vi "Automated JV Measurement.vi"() -> ()   [LabVIEW 2011]
uses:
  TypeDefs/Scan settings.ctl
  TypeDefs/Settings Boolean.ctl
  TypeDefs/State Enumerate Ring.ctl
  <vilib>/Utility/file.llb/Write To Spreadsheet File (string).vi
  <vilib>/Utility/file.llb/Write To Spreadsheet File (DBL).vi
  <instrlib>/keithley_24xx/Keithley 24XX/Keithley 24XX.lvlib
panel:
  in  "Intensity/EQE off":bool
  out "Scan stopped?":bool
  out "Max P cond. cont. Lab.txt array":string[](array[string])
  out "Max P cont. Lab.txt array":string[](array[string])
  out "J-t cont. Lab.txt array":string[](array[string])
  out "J-V cond. cont. Lab.txt array":string[](array[string])
  out "J-V cont. Lab.txt array":string[](array[string])
  out "Go to neg. lim. Lab.txt array":string[](array[string])
  out "Start scan Lab.txt array":string[](array[string])
  out "Init/idle Lab.txt array":string[](array[string])
  out "Measure Lab.txt array":string[](array[string])
  out "Sample set. Lab.txt array":string[](array[string])
  out "Scan set. Lab.txt array":string[](array[string])
  out "Advanced Lab.txt array":string[](array[string])
  out "Calibrate?":bool
  out "reference (out) 4":i32=4168
  out "reference (out) 3":i32=4168
  out "reference (out) 2":i32=4168
  out "reference (out)":i32=4168
  out "Abort":bool
  in  "Tab Control":T1(tab)
  in  "Manual mode":bool
  in  "Cell Settings Array 1":T2(array[cluster])=[{"Cell Position"=1, "Cell Label"="", "Pixel to measure"=0, "Area (cm^2)"=0.0935, "Variable"="", "Variable value"="", "Scan settings in queue"=0}, {"Cell Position"=2, "Cell Label"="", "Pixel to measure"=0, "Area (cm^2)"=0.0935, "Variable"="", "Variable value"="", "Scan settings in queue"=0}, {"Cell Position"=3, "Cell Label"="", "Pixel to measure"=0, "Area (cm^2)"=0.0935, "Variable"="", "Variable value"="", "Scan settings in queue"=0}, {"Cell Position"=4, "Cell Label"="", "Pixel to measure"=0, "Area (cm^2)"=0.0935, "Variable"="", "Variable value"="", "Scan settings in queue"=0}, {"Cell Position"=5, "Cell Label"="", "Pixel to measure"=0, "Area (cm^2)"=0.0935, "Variable"="", "Variable value"="", "Scan settings in queue"=0}, {"Cell Position"=6, "Cell Label"="", "Pixel to measure"=0, "Area (cm^2)"=0.0935, "Variable"="", "Variable value"="", "Scan settings in queue"=0}, {"Cell Position"=7, "Cell Label"="", "Pixel to measure"=0, "Area (cm^2)"=0.0935, "Variable"="", "Variable value"="", "Scan settings in queue"=0}, {"Cell Position"=8, "Cell Label"="", "Pixel to measure"=0, "Area (cm^2)"=0.0935, "Variable"="", "Variable value"="", "Scan settings in queue"=0}, {"Cell Position"=9, "Cell Label"="", "Pixel to measure"=0, "Area (cm^2)"=0.0935, "Variable"="", "Variable value"="", "Scan settings in queue"=0}, {"Cell Position"=10, "Cell Label"="", "Pixel to measure"=0, "Area (cm^2)"=0.0935, "Variable"="", "Variable value"="", "Scan settings in queue"=0}, {"Cell Position"=11, "Cell Label"="", "Pixel to measure"=0, "Area (cm^2)"=0.0935, "Variable"="", "Variable value"="", "Scan settings in queue"=0}, {"Cell Position"=12, "Cell Label"="", "Pixel to measure"=0, "Area (cm^2)"=0.0935, "Variable"="", "Variable value"="", "Scan settings in queue"=0}, {"Cell Position"=13, "Cell Label"="", "Pixel to measure"=0, "Area (cm^2)"=0.0935, "Variable"="", "Variable value"="", "Scan settings in queue"=0}, {"Cell Position"=14, "Cell Label"="", "Pixel to measure"=0, "Area (cm^2)"=0.0935, "Variable"="", "Variable value"="", "Scan settings in queue"=0}, {"Cell Position"=15, "Cell Label"="", "Pixel to measure"=0, "Area (cm^2)"=0.0935, "Variable"="", "Variable value"="", "Scan settings in queue"=0}, {"Cell Position"=16, "Cell Label"="", "Pixel to measure"=0, "Area (cm^2)"=0.0935, "Variable"="", "Variable value"="", "Scan settings in queue"=0}] {"Scan settings in queue" items=["Default_Inv", "Default_Std", "Solarprint", "StandardJV", "TEST_std", "Test_Manual_JV_Jt_mppt", "Test_inv", "Test_inv2", "Test_inv3", "Test_inv4", "Test_inv_mpp", "Test_inv_mppt", "Test_inv_mppt_Jt", "Test_std_2", "Test_std_3", "Test_std_4", "Test_std_5"]; "Pixel to measure" items=["All", "1", "2", "3", "4", "5", "6", "7", "8"]}
  in  "Load details from file":bool
  in  "Save details to file":bool
  out "X-Y stage controller":bool
  out "PCB controller":bool
  out "Keithley 2400":bool
  in  "User Name":string
  in  "Experiment Title":string
  out "Status:":string
  in  "Move to load pos.":bool
  in  "Exit":bool
  out "Arduino":bool
  in  "Update":bool
  in  "Scan settings":T3={"J-V scan"=TRUE, "J-t scan"=FALSE, "Min voltage (V)"=0.0, "Max voltage (V)"=1.4, "Step (V)"=0.01, "Measurement delay (ms)"=10.0, "1st scan FB-SC"=TRUE, "Inverted structure"=FALSE, "Stabilisation time (s)"=0.0, "Stabilisation mode"=0, "Stabilisation value (V or A) "=0.0, "Step time (s)"=1.0, "Integration time"=0, "Repeat light scans"=FALSE, "Stabilisation in the dark?"=FALSE, "J-t Min (V)"=0.0, "J-t Max (V)"=1.4, "J-t Step (V)"=0.01, "Max. power stabilisation"=FALSE, "J-t 1st scan FB-SC"=TRUE, "J-t Inverted structure"=FALSE, "Max power tracking"=FALSE, "Vmp (V)"=0.7, "Total stabilisation time (s)"=100.0, "J-t best pixel only"=7, "Max power best pixel only"=7, "Vmp from J-V scan"=FALSE, "Intensity dependence"=FALSE, "P dep best pixel only"=7, "External quantum efficiency"=FALSE, "EQE best pixel only"=7, "WL min (nm)"=300.0, "WL max (nm)"=900.0, "WL step (nm)"=5.0, "Wait (ms)"=100.0, "No. of repeat scans"=2.0, "Only repeat for best pixel"=7, "Chopper Freq. min (Hz)"=90.0, "Time Constant min (s)"=2.0, "Stabilisation time step (s)"=1.0, "Illumination conditions"=2, "Scan rate min (V/s)"=0.1, "Scan rate max (V/s)"=1.0, "No. of scan rate steps"=1.0, "Scan rate voltage step priority"=FALSE, "Scan rate measurement delay priority"=FALSE, "J-t Illumination conditions"=0, "Chopper Freq. max (Hz)"=200.0, "No. of freq. steps"=1.0, "Time Constant max (s)"=2.0, "No. of t const. steps"=1.0, "White bias min (no. of suns)"=0.1, "White bias max (no. of suns)"=1.0, "No. of white bias steps"=1.0, "Repeat EQE scans"=FALSE, "No. of EQE scans"=2.0, "Max P stab. Specific voltage"=FALSE} {"No. of EQE scans" min=1.0 step=1.0; "No. of white bias steps" min=1.0 step=1.0; "No. of t const. steps" min=1.0 step=1.0; "Time Constant max (s)" items=["0.01s", "0.03s", "0.1s", "0.3s", "1s", "3s"]; "No. of freq. steps" min=1.0 step=1.0; "J-t Illumination conditions" items=["Light only", "Dark only", "Light then dark", "Dark then light"]; "No. of scan rate steps" min=1.0 step=1.0; "Illumination conditions" items=["Light only", "Dark only", "Light then dark", "Dark then light", "Light then dark then light", "Dark then light then dark"]; "Time Constant min (s)" items=["0.01s", "0.03s", "0.1s", "0.3s", "1s", "3s"]; "Only repeat for best pixel" items=["only for best pixel", "for best 2 pixels", "for best 3 pixels", "for best 4 pixels", "for best 5 pixels", "for best 6 pixels", "for best 7 pixels", "for all pixels"]; "No. of repeat scans" min=1.0 step=1.0; "EQE best pixel only" items=["only the best pixel", "the best 2 pixel", "the best 3 pixel", "the best 4 pixel", "the best 5 pixel", "the best 6 pixel", "the best 7 pixel", "all pixels"]; "P dep best pixel only" items=["only the best pixel", "the best 2 pixels", "the best 3 pixels", "the best 4 pixels", "the best 5 pixels", "the best 6 pixels", "the best 7 pixels", "all pixels"]; "Max power best pixel only" items=["only the best pixel", "the best 2 pixels", "the best 3 pixels", "the best 4 pixels", "the best 5 pixels", "the best 6 pixels", "the best 7 pixels", "all pixels"]; "J-t best pixel only" items=["only the best pixel", "the best 2 pixels", "the best 3 pixels", "the best 4 pixels", "the best 5 pixels", "the best 6 pixels", "the best 7 pixels", "all pixels"]; "Integration time" items=["Fast", "Normal", "High Accuracy"]; "Stabilisation mode" items=["V", "I"]; "Measurement delay (ms)" min=10.0}
  in  "Save New Settings As...":string
  in  "Check Saved Settings":u16(ring) items=["Default_Inv", "Default_Std", "Solarprint", "StandardJV", "TEST_std", "Test_Manual_JV_Jt_mppt", "Test_inv", "Test_inv2", "Test_inv3", "Test_inv4", "Test_inv_mpp", "Test_inv_mppt", "Test_inv_mppt_Jt", "Test_std_2", "Test_std_3", "Test_std_4", "Test_std_5"]
  in  "Save new settings":bool
  in  "Delete settings":bool
  out "Measurement status:":string
  out "Log Table":string[][](table)
  out "JV Curve":cluster{"Y":dbl[], "Y":dbl[]}[](graph)
  out "Number of suns":string
  in  "Stop Scan 2":bool
  in  "Start Scan":bool
  out "Finish time":timestamp caption="This experiment will finish at approximately" format="%<%H:%M:%S   %d/%m/%y>T"
  out "Time left":dbl caption="You have" format="%<%H:%M:%S>t"
  out "Measurement queue":T5(array[cluster]) {"Pixel to measure" items=["All", "1", "2", "3", "4", "5", "6", "7", "8"]}
  out "Current Angle (degrees)":dbl
  out "Pin":dbl
  out "Current (A)":dbl
  in  "Pixel":i64
  in  "Cell":i64
  in  "Shutter closed":bool
  in  "Shutter open":bool
  in  "error in (no error) 3":errorcluster
  in  "Set diode pos":bool
  in  "Go to negative limit":bool
  out "Y position":string
  out "X position":string
  in  "X -ve":bool
  in  "X +ve":bool
  in  "Y -ve":bool
  in  "Y +ve":bool
  in  "Change pin on pcb":bool
  in  "Measure current":bool
  out "File path for master log":path
  out "Experiment type":u16(ring) items=["PCB-Keithley", "PCB-EQE", "Manual-Keithley", "Manual-EQE"]
  # "Cell #"
  # "Label"
  # "Pixel #"
  # "Area (cm^2)"
  # "Variable"
  # "Variable Value"
  # "Scan Settings"
  # "Connected instruments"
  # "Label"
  # "Pixel"
  # "Condition"
  # "Jsc"
  # "Voc"
  # "PCE"
  # "FF"
  # "Vmp"
  # "to work on something else."
  # "Position"
  # "Label"
  # "Pixel"
  # "Area"
  # "Variable"
  # "Variable Value"
  # "Scan Settings"
  # "Condition"
  # "Measurement Type"
  # "Pixel Selection"
  # "Motor Control"
  # "Filter Wheel"
  # "Shutter Control"
  # "Switch board configuration"
  # "Current Measurement"
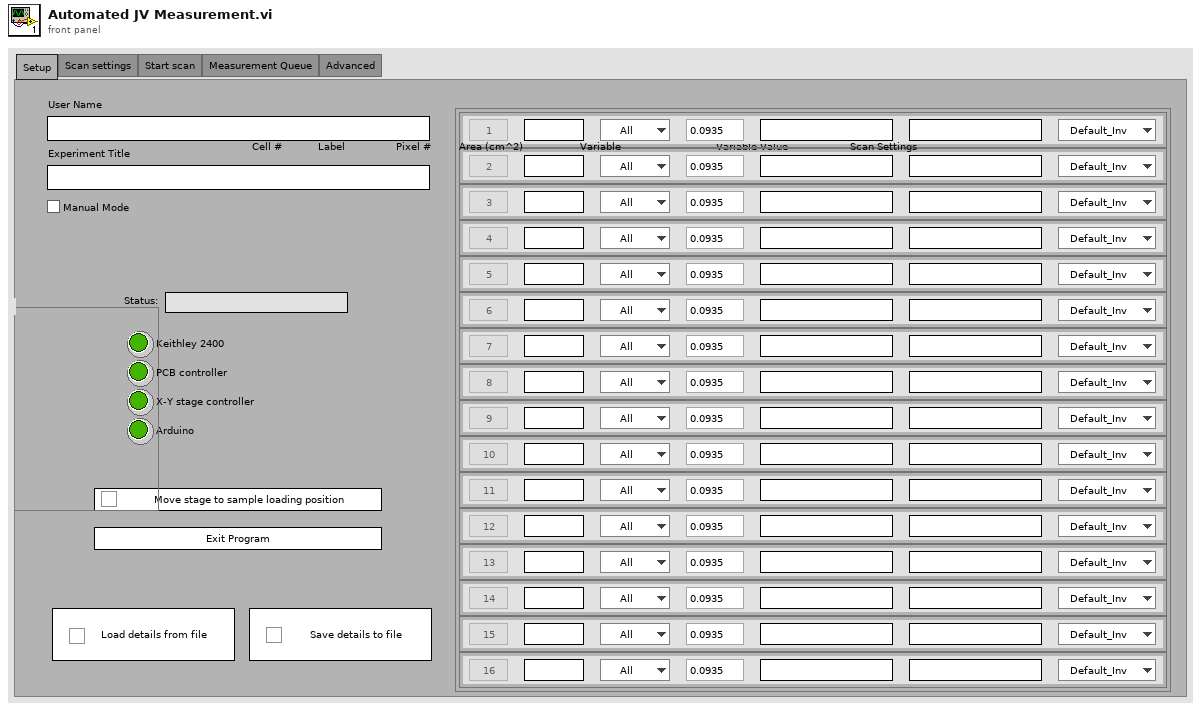
[diagram p1: front panel]
types:
  T1 = enum32{"Setup", "Scan settings", "Start scan", "Measurement Queue", "Advanced"}
  T2 = cluster{"Cell Position":i32, "Cell Label":string, "Pixel to measure":u16, "Area (cm^2)":dbl, "Variable":string, "Variable value":string, "Scan settings in queue":u16}[]
  T3 = typedef "Scan settings.ctl" = cluster{"J-V scan":T4, "J-t scan":bool, "Min voltage (V)":dbl, "Max voltage (V)":dbl, "Step (V)":dbl, "Measurement delay (ms)":dbl, "1st scan FB-SC":bool, "Inverted structure":bool, "Stabilisation time (s)":dbl, "Stabilisation mode":u16, "Stabilisation value (V or A) ":dbl, "Step time (s)":dbl, "Integration time":u16, "Repeat light scans":bool, "Stabilisation in the dark?":bool, "J-t Min (V)":dbl, "J-t Max (V)":dbl, "J-t Step (V)":dbl, "Max. power stabilisation":bool, "J-t 1st scan FB-SC":bool, "J-t Inverted structure":bool, "Max power tracking":bool, "Vmp (V)":dbl, "Total stabilisation time (s)":dbl, "J-t best pixel only":u16, "Max power best pixel only":u16, "Vmp from J-V scan":bool, "Intensity dependence":bool, "P dep best pixel only":u16, "External quantum efficiency":bool, "EQE best pixel only":u16, "WL min (nm)":dbl, "WL max (nm)":dbl, "WL step (nm)":dbl, "Wait (ms)":dbl, "No. of repeat scans":dbl, "Only repeat for best pixel":u16, "Chopper Freq. min (Hz)":dbl, "Time Constant min (s)":dbl, "Stabilisation time step (s)":dbl, "Illumination conditions":u16, "Scan rate min (V/s)":dbl, "Scan rate max (V/s)":dbl, "No. of scan rate steps":dbl, "Scan rate voltage step priority":bool, "Scan rate measurement delay priority":bool, "J-t Illumination conditions":u16, "Chopper Freq. max (Hz)":dbl, "No. of freq. steps":dbl, "Time Constant max (s)":dbl, "No. of t const. steps":dbl, "White bias min (no. of suns)":dbl, "White bias max (no. of suns)":dbl, "No. of white bias steps":dbl, "Repeat EQE scans":bool, "No. of EQE scans":dbl, "Max P stab. Specific voltage":bool}
  T4 = typedef "Settings Boolean.ctl" = bool
  T5 = cluster{"Cell Position":i32, "Cell Label":string, "Pixel to measure":u16, "Area (cm^2)":dbl, "Variable":string, "Variable value":string, "Scan settings in queue":u16, "Light or dark":string, "Measurement type":string}[]
  T6 = typedef "State Enumerate Ring.ctl" = enum16{"Initialise", "Idle", "Measure", "Notify"}
  T7 = enum8{"Enabled", "Disabled", "Disabled and Grayed Out"}
  T8 = enum16{"Left Button", "Center Button", "Right Button", "Window Close"}
  T9 = cluster{"Cell Position":i32, "Cell Label":string, "Pixel to measure":u16, "Area (cm^2)":dbl, "Variable":string, "Variable value":string, "Scan settings in queue":u16, "Light or dark":string, "Measurement type":string}
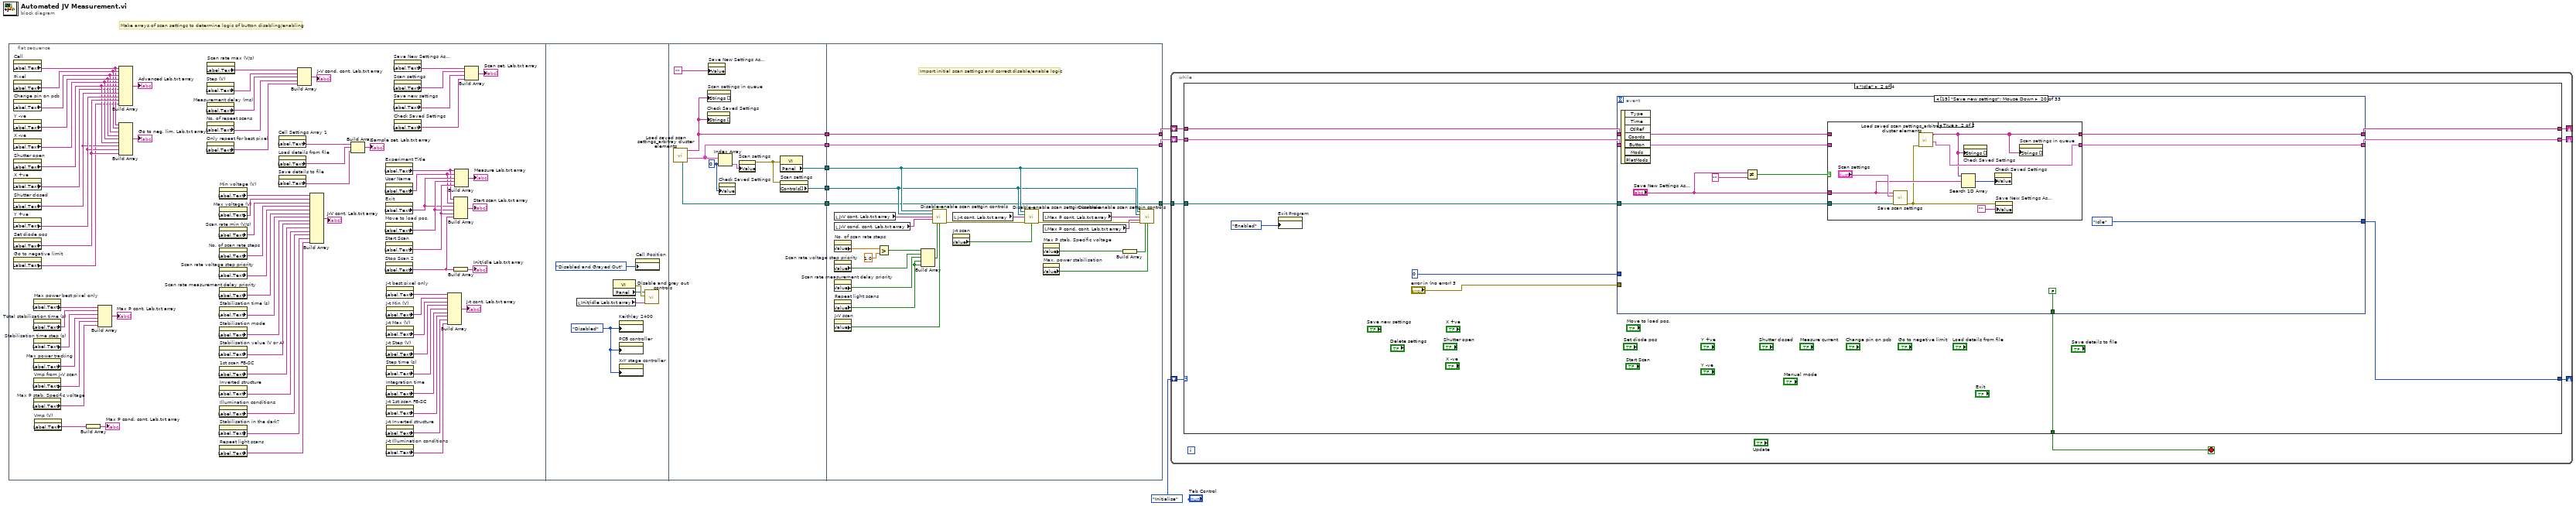
[diagram p0: block diagram]
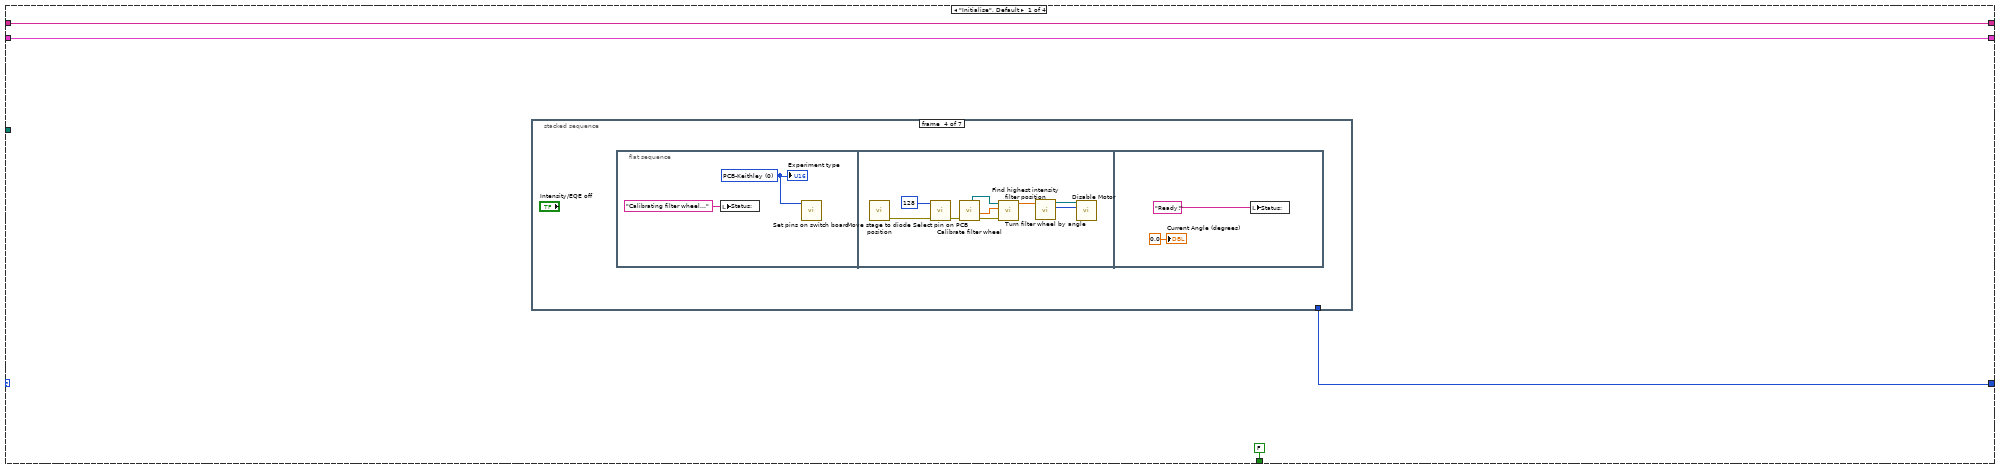
[diagram p2: hidden frame]
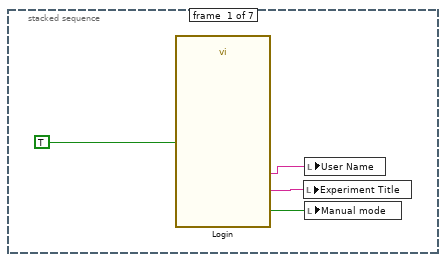
[diagram p3: hidden frame]
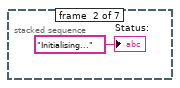
[diagram p4: hidden frame]
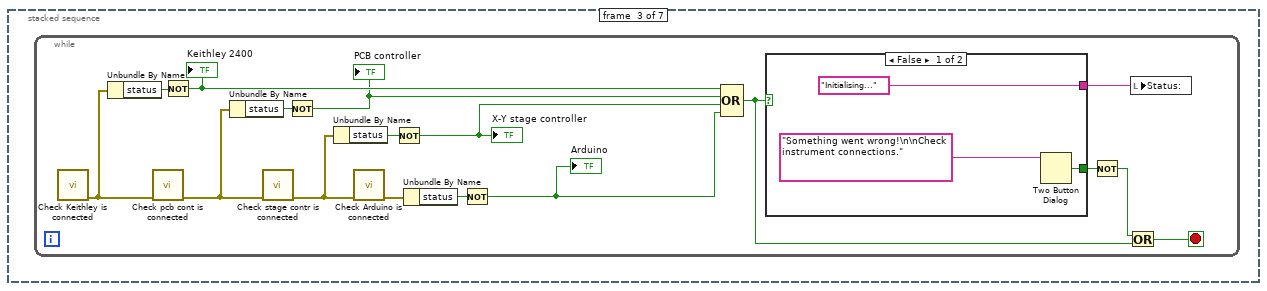
[diagram p5: hidden frame]
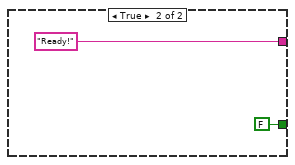
[diagram p6: hidden frame]
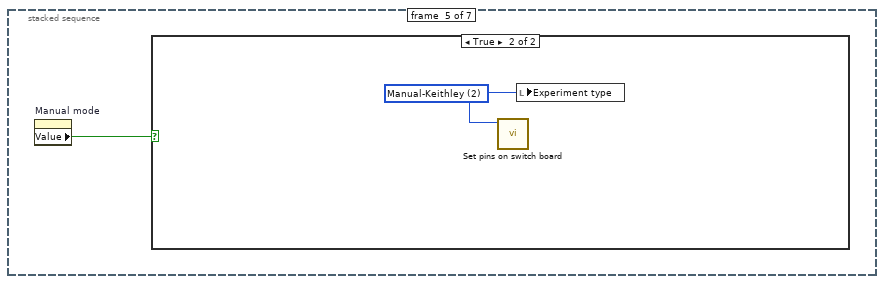
[diagram p7: hidden frame]
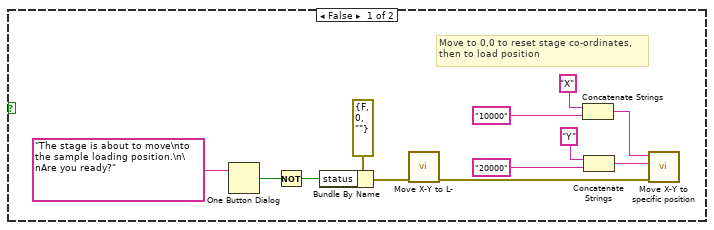
[diagram p8: hidden frame]
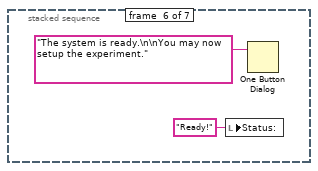
[diagram p9: hidden frame]
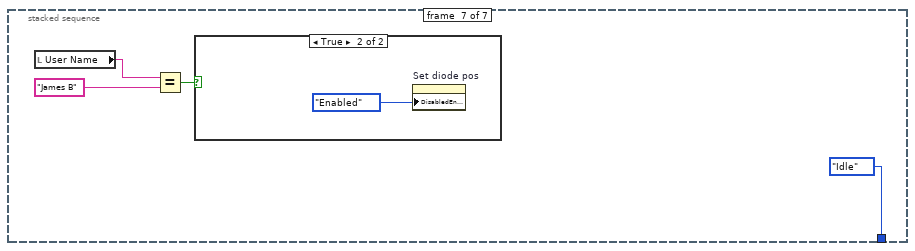
[diagram p10: hidden frame]
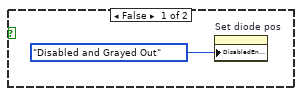
[diagram p11: hidden frame]
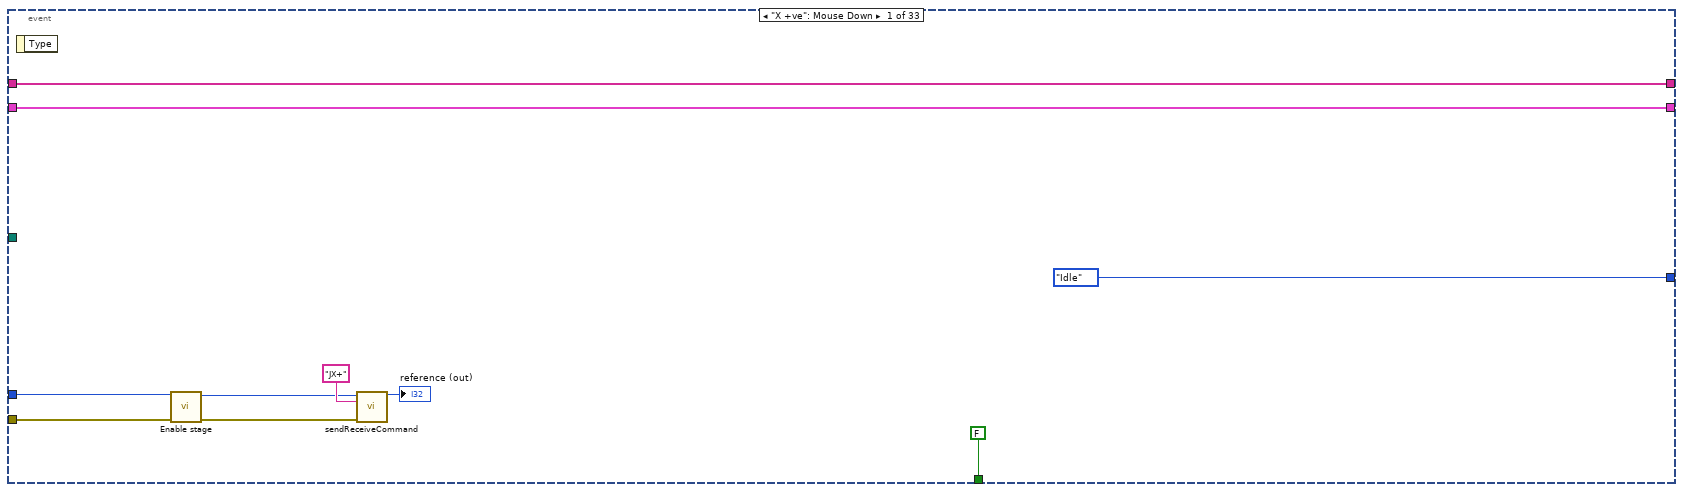
[diagram p12: hidden frame]
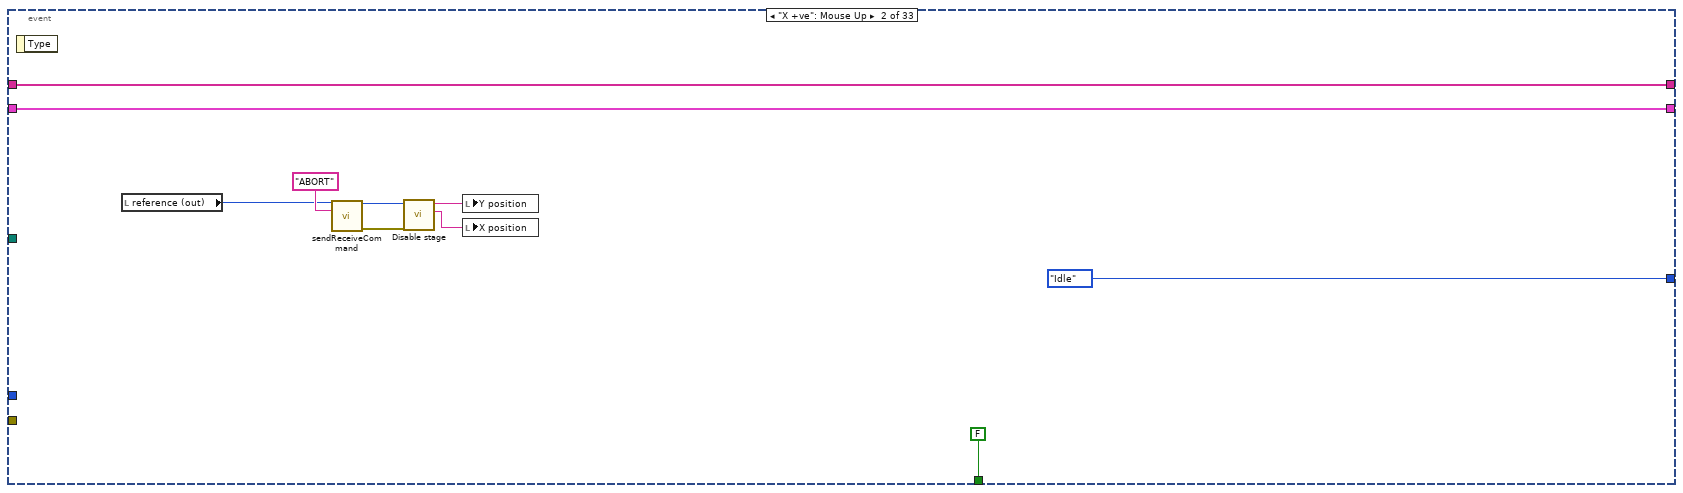
[diagram p13: hidden frame]
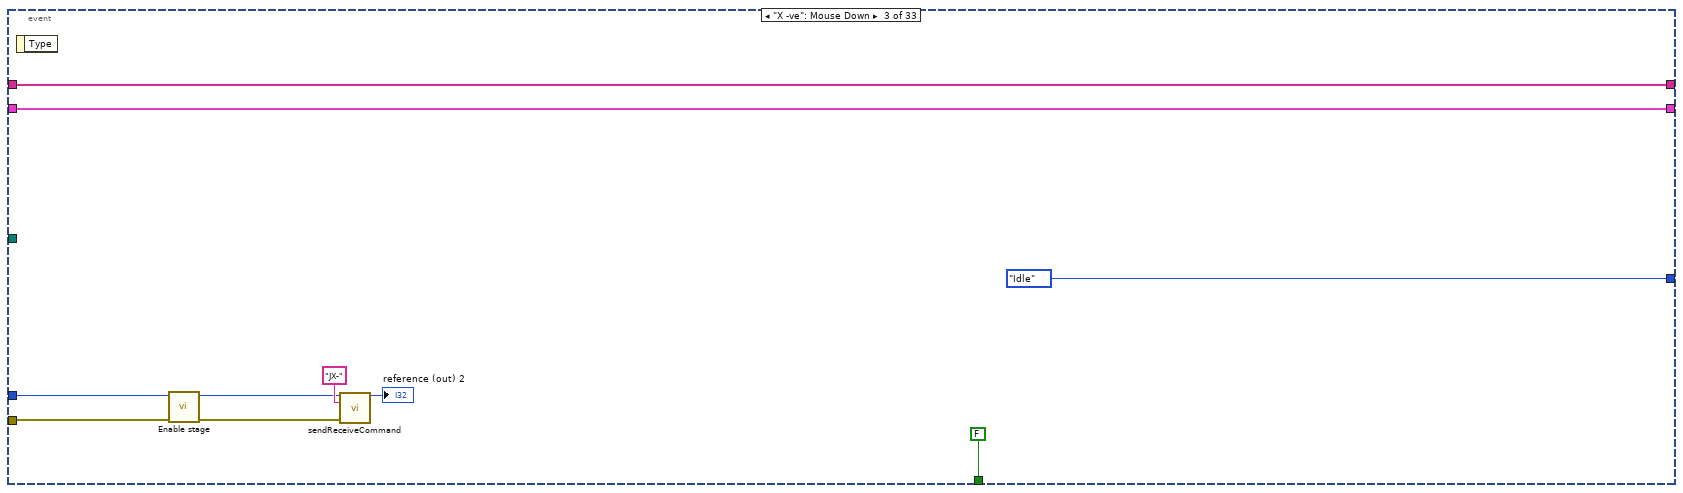
[diagram p14: hidden frame]
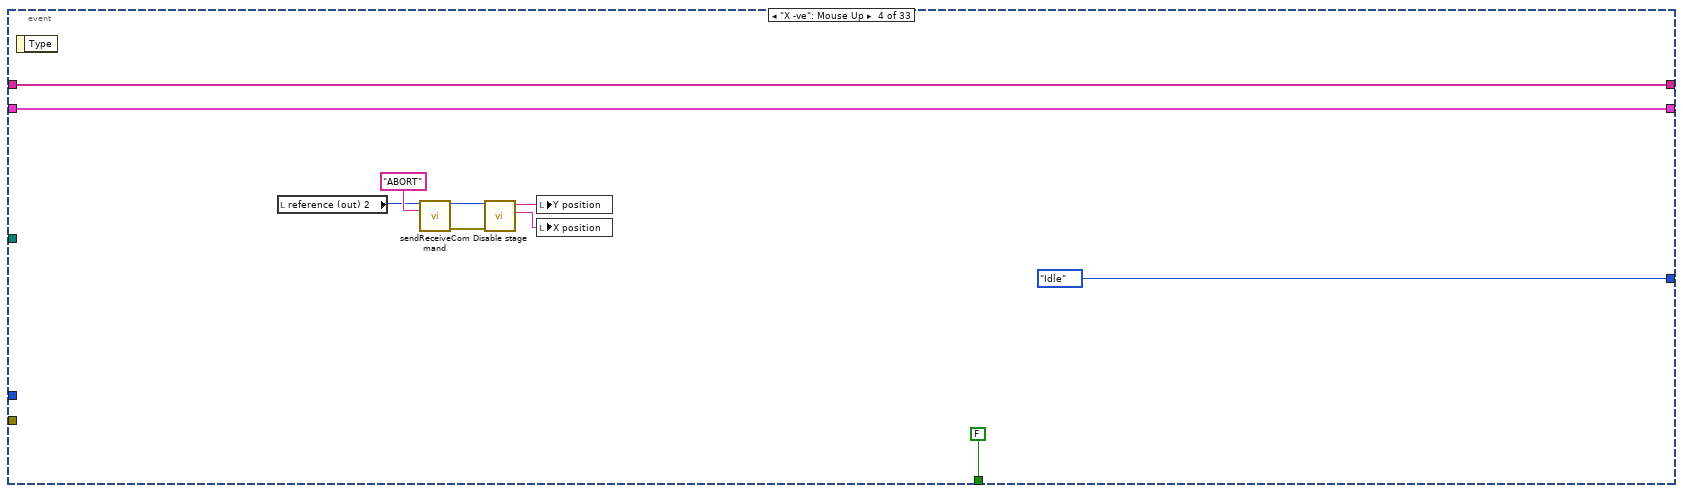
[diagram p15: hidden frame]
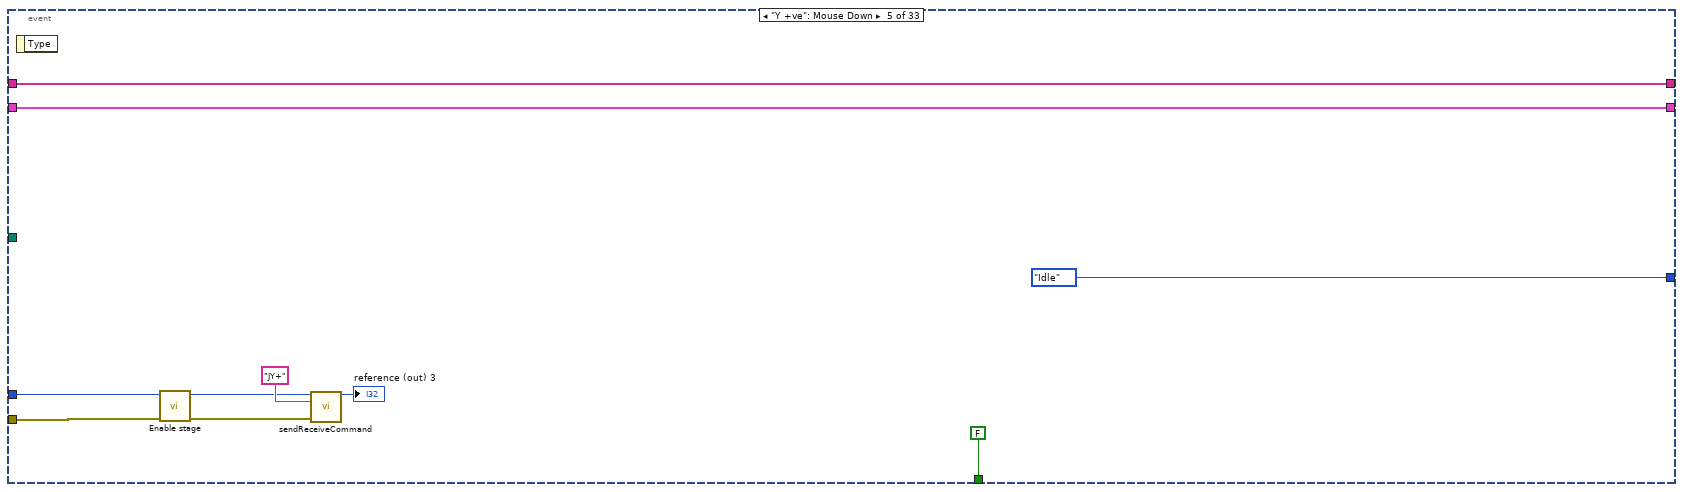
[diagram p16: hidden frame]
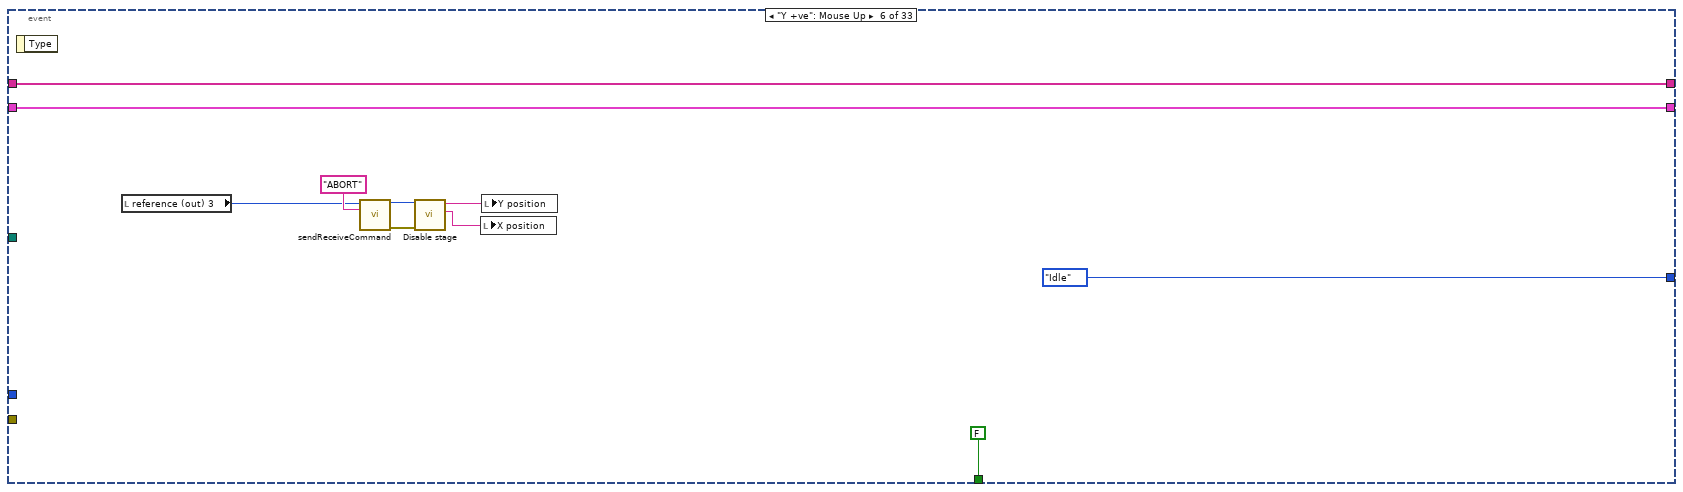
[diagram p17: hidden frame]
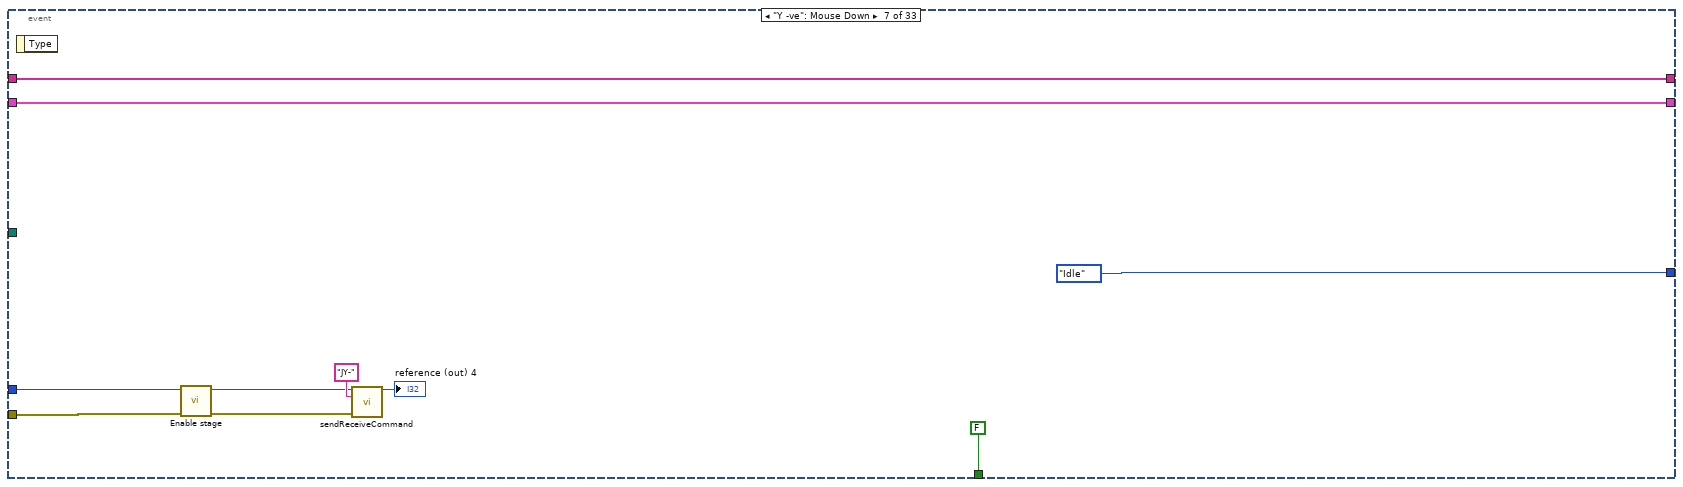
[diagram p18: hidden frame]
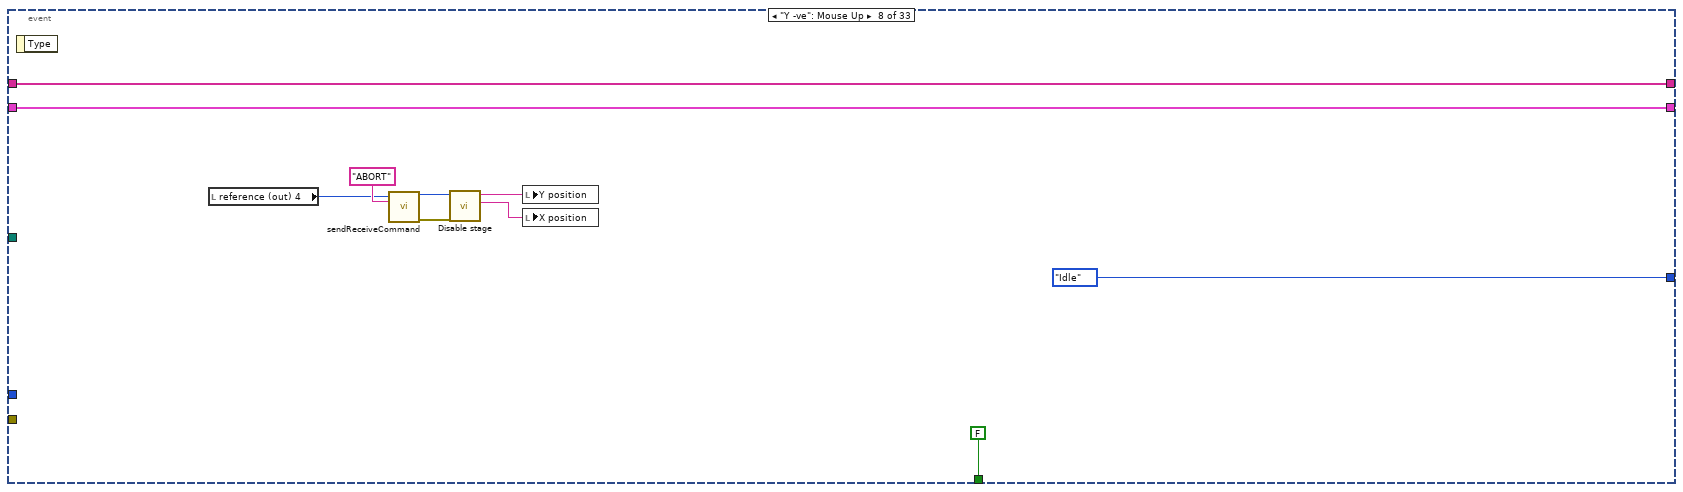
[diagram p19: hidden frame]
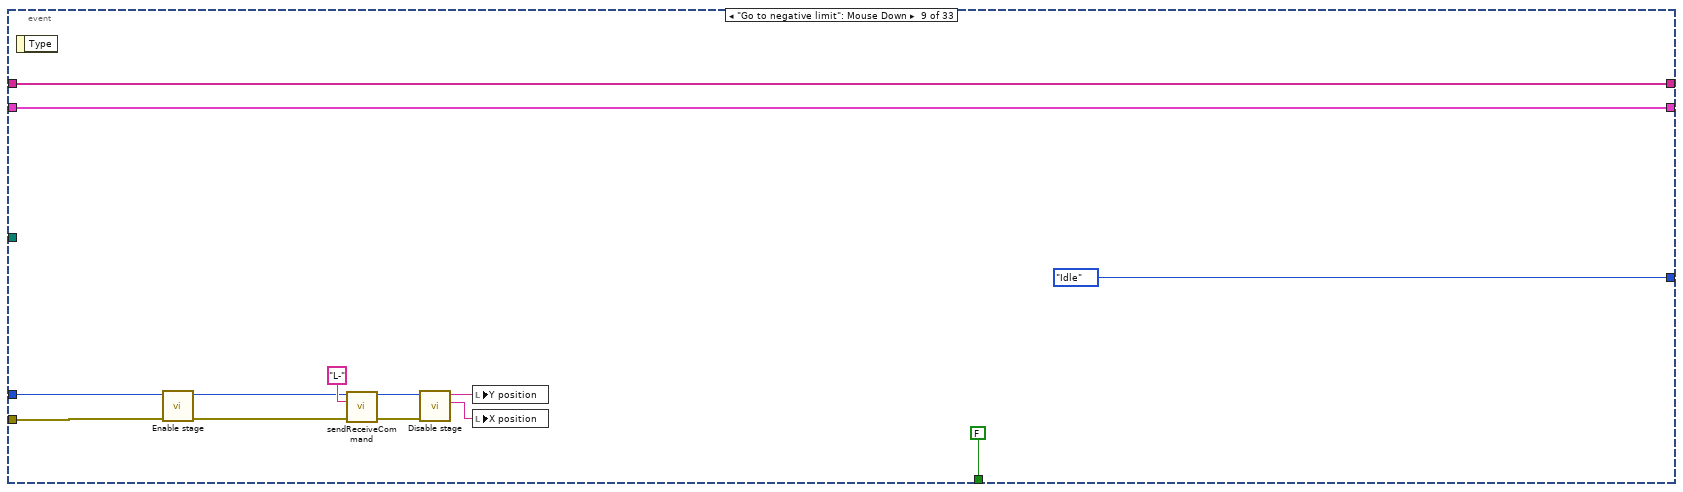
[diagram p20: hidden frame]
diagram:
  # "Make arrays of scan settings to determine logic of button disabling/enabling"
  n1 = flat-sequence {
    tunnel: [w94] -> w8
    tunnel: [w92] -> w7
    tunnel: [w90] -> w6
    tunnel: [w88] -> w5
    tunnel: [w87] -> w4
    tunnel: w8 -> [w97]
    tunnel: w7 -> [w95]
    tunnel: w6 -> [w96]
    tunnel: w5 -> [w99]
    tunnel: w4 -> [w98]
    tunnel: [w97] -> w3
    tunnel: [w96] -> w2
    tunnel: [w95] -> w1
    frame #0 {
      n2 = property on="Cell" class="DigNum (strict)"() -> ("Label.Text"=w32:string)  [unwired: 2 in, 2 out]
      n3 = property on="Pixel" class="DigNum (strict)"() -> ("Label.Text"=w33:string)  [unwired: 2 in, 2 out]
      n4 = property on="Change pin on pcb" class="Bool (strict)"() -> ("Label.Text"=w34:string)  [unwired: 2 in, 2 out]
      n5 = property on="Y -ve" class="Bool (strict)"() -> ("Label.Text"=w35:string)  [unwired: 2 in, 2 out]
      n6 = property on="X -ve" class="Bool (strict)"() -> ("Label.Text"=w36:string)  [unwired: 2 in, 2 out]
      n7 = property on="Shutter open" class="Bool (strict)"() -> ("Label.Text"=w37:string)  [unwired: 2 in, 2 out]
      n8 = property on="X +ve" class="Bool (strict)"() -> ("Label.Text"=w29:string)  [unwired: 2 in, 2 out]
      n9 = property on="Shutter closed" class="Bool (strict)"() -> ("Label.Text"=w38:string)  [unwired: 2 in, 2 out]
      n10 = property on="Y +ve" class="Bool (strict)"() -> ("Label.Text"=w39:string)  [unwired: 2 in, 2 out]
      n11 = property on="Set diode pos" class="Bool (strict)"() -> ("Label.Text"=w40:string)  [unwired: 2 in, 2 out]
      n12 = property on="Go to negative limit" class="Bool (strict)"() -> ("Label.Text"=w30:string)  [unwired: 2 in, 2 out]
      n13 = property on="Max power best pixel only" class="Ring (strict)"() -> ("Label.Text"=w20:string)  [unwired: 2 in, 2 out]
      n14 = property on="Total stabilisation time (s)" class="DigNum (strict)"() -> ("Label.Text"=w21:string)  [unwired: 2 in, 2 out]
      n15 = property on="Stabilisation time step (s)" class="DigNum (strict)"() -> ("Label.Text"=w22:string)  [unwired: 2 in, 2 out]
      n16 = property on="Max power tracking" class="Bool (strict)"() -> ("Label.Text"=w23:string)  [unwired: 2 in, 2 out]
      n17 = property on="Vmp from J-V scan" class="Bool (strict)"() -> ("Label.Text"=w24:string)  [unwired: 2 in, 2 out]
      n18 = property on="Max P stab. Specific voltage" class="Bool (strict)"() -> ("Label.Text"=w25:string)  [unwired: 2 in, 2 out]
      n19 = property on="Vmp (V)" class="DigNum (strict)"() -> ("Label.Text"=w27:string)  [unwired: 2 in, 2 out]
      n20 = Build Array(w27) -> (→"Max P cond. cont. Lab.txt array":string[])
      n21 = Build Array(w20, w21, w22, w23, w24, w25) -> (→"Max P cont. Lab.txt array":string[])
      n22 = Build Array(w32, w33, w34, w35, w36, w37, w29, w38, w39, w40, w30) -> (→"Advanced Lab.txt array":string[])
      n23 = Build Array(w32, w33, w34, w35, w36, w37, w38, w39, w40) -> (→"Go to neg. lim. Lab.txt array":string[])
      n24 = property on="Step (V)" class="DigNum (strict)"() -> ("Label.Text"=w75:string)  [unwired: 2 in, 2 out]
      n25 = property on="Measurement delay (ms)" class="DigNum (strict)"() -> ("Label.Text"=w76:string)  [unwired: 2 in, 2 out]
      n26 = property on="No. of repeat scans" class="DigNum (strict)"() -> ("Label.Text"=w77:string)  [unwired: 2 in, 2 out]
      n27 = property on="Only repeat for best pixel" class="Ring (strict)"() -> ("Label.Text"=w78:string)  [unwired: 2 in, 2 out]
      n28 = property on="Scan rate max (V/s)" class="DigNum (strict)"() -> ("Label.Text"=w80:string)  [unwired: 2 in, 2 out]
      n29 = property on="Min voltage (V)" class="DigNum (strict)"() -> ("Label.Text"=w60:string)  [unwired: 2 in, 2 out]
      n30 = property on="Max voltage (V)" class="DigNum (strict)"() -> ("Label.Text"=w61:string)  [unwired: 2 in, 2 out]
      n31 = property on="Scan rate min (V/s)" class="DigNum (strict)"() -> ("Label.Text"=w62:string)  [unwired: 2 in, 2 out]
      n32 = property on="No. of scan rate steps" class="DigNum (strict)"() -> ("Label.Text"=w63:string)  [unwired: 2 in, 2 out]
      n33 = property on="Scan rate voltage step priority" class="Bool (strict)"() -> ("Label.Text"=w64:string)  [unwired: 2 in, 2 out]
      n34 = property on="Scan rate measurement delay priority" class="Bool (strict)"() -> ("Label.Text"=w65:string)  [unwired: 2 in, 2 out]
      n35 = property on="Stabilisation time (s)" class="DigNum (strict)"() -> ("Label.Text"=w66:string)  [unwired: 2 in, 2 out]
      n36 = property on="Stabilisation mode" class="Ring (strict)"() -> ("Label.Text"=w67:string)  [unwired: 2 in, 2 out]
      n37 = property on="Stabilisation value (V or A)" class="DigNum (strict)"() -> ("Label.Text"=w68:string)  [unwired: 2 in, 2 out]
      n38 = property on="1st scan FB-SC" class="Bool (strict)"() -> ("Label.Text"=w69:string)  [unwired: 2 in, 2 out]
      n39 = property on="Inverted structure" class="Bool (strict)"() -> ("Label.Text"=w70:string)  [unwired: 2 in, 2 out]
      n40 = property on="Illumination conditions" class="Ring (strict)"() -> ("Label.Text"=w71:string)  [unwired: 2 in, 2 out]
      n41 = property on="Stabilisation in the dark?" class="Bool (strict)"() -> ("Label.Text"=w72:string)  [unwired: 2 in, 2 out]
      n42 = property on="Repeat light scans" class="Bool (strict)"() -> ("Label.Text"=w73:string)  [unwired: 2 in, 2 out]
      n43 = property on="Cell Settings Array 1" class="Arr (strict)"() -> ("Label.Text"=w47:string)  [unwired: 2 in, 2 out]
      n44 = property on="Load details from file" class="Bool (strict)"() -> ("Label.Text"=w48:string)  [unwired: 2 in, 2 out]
      n45 = property on="Save details to file" class="Bool (strict)"() -> ("Label.Text"=w49:string)  [unwired: 2 in, 2 out]
      n46 = Build Array(w80, w75, w76, w77, w78) -> (→"J-V cond. cont. Lab.txt array":string[])
      n47 = Build Array(w60, w61, w62, w63, w64, w65, w66, w67, w68, w69, w70, w71, w72, w73) -> (→"J-V cont. Lab.txt array":string[])
      n48 = Build Array(w47, w48, w49) -> (→"Sample set. Lab.txt array":string[])
      n49 = property on="Experiment Title" class="Str"() -> ("Label.Text"=w53:string)  [unwired: 2 in, 2 out]
      n50 = property on="User Name" class="Str"() -> ("Label.Text"=w54:string)  [unwired: 2 in, 2 out]
      n51 = property on="Exit" class="Bool (strict)"() -> ("Label.Text"=w55:string)  [unwired: 2 in, 2 out]
      n52 = property on="Move to load pos." class="Bool (strict)"() -> ("Label.Text"=w56:string)  [unwired: 2 in, 2 out]
      n53 = property on="Start Scan" class="Bool (strict)"() -> ("Label.Text"=w57:string)  [unwired: 2 in, 2 out]
      n54 = property on="Stop Scan 2" class="Bool"() -> ("Label.Text"=w59:string)  [unwired: 2 in, 2 out]
      n55 = property on="J-t best pixel only" class="Ring (strict)"() -> ("Label.Text"=w10:string)  [unwired: 2 in, 2 out]
      n56 = property on="J-t Min (V)" class="DigNum (strict)"() -> ("Label.Text"=w11:string)  [unwired: 2 in, 2 out]
      n57 = property on="J-t Max (V)" class="DigNum (strict)"() -> ("Label.Text"=w12:string)  [unwired: 2 in, 2 out]
      n58 = property on="J-t Step (V)" class="DigNum (strict)"() -> ("Label.Text"=w13:string)  [unwired: 2 in, 2 out]
      n59 = property on="Step time (s)" class="DigNum (strict)"() -> ("Label.Text"=w14:string)  [unwired: 2 in, 2 out]
      n60 = property on="Integration time" class="Ring (strict)"() -> ("Label.Text"=w15:string)  [unwired: 2 in, 2 out]
      n61 = property on="J-t 1st scan FB-SC" class="Bool (strict)"() -> ("Label.Text"=w16:string)  [unwired: 2 in, 2 out]
      n62 = property on="J-t Inverted structure" class="Bool (strict)"() -> ("Label.Text"=w17:string)  [unwired: 2 in, 2 out]
      n63 = property on="J-t Illumination conditions" class="Ring (strict)"() -> ("Label.Text"=w18:string)  [unwired: 2 in, 2 out]
      n64 = property on="Save New Settings As..." class="Str"() -> ("Label.Text"=w42:string)  [unwired: 2 in, 2 out]
      n65 = property on="Scan settings" class="Clust (strict)"() -> ("Label.Text"=w43:string)  [unwired: 2 in, 2 out]
      n66 = property on="Save new settings" class="Bool (strict)"() -> ("Label.Text"=w44:string)  [unwired: 2 in, 2 out]
      n67 = property on="Check Saved Settings" class="Ring (strict)"() -> ("Label.Text"=w45:string)  [unwired: 2 in, 2 out]
      n68 = Build Array(w10, w11, w12, w13, w14, w15, w16, w17, w18) -> (→"J-t cont. Lab.txt array":string[])
      n69 = Build Array(w53, w54, w55, w56, w57, w59) -> (→"Start scan Lab.txt array":string[])
      n70 = Build Array(w59) -> (→"Init/idle Lab.txt array":string[])
      n71 = Build Array(w53, w54, w55, w56, w57) -> (→"Measure Lab.txt array":string[])
      n72 = Build Array(w42, w43, w44, w45) -> (→"Scan set. Lab.txt array":string[])
    }
    frame #1 {
      w81 = T7."Disabled" ("Disabled")
      n73 = local read "Init/idle Lab.txt array"() -> (w85:string[])
      n74 = property class="VI"() -> (error out=w84:errorcluster, "Panel"=w83:refnum<vi>)  [unwired: 2 in, 1 out]
      n75 = property on="Keithley 2400" class="Bool (strict)"("DisabledEnum"=w81) -> ()  [unwired: 2 in, 2 out]
      n76 = property on="PCB controller" class="Bool (strict)"("DisabledEnum"=w81) -> ()  [unwired: 2 in, 2 out]
      n77 = property on="X-Y stage controller" class="Bool (strict)"("DisabledEnum"=w81) -> ()  [unwired: 2 in, 2 out]
      n78 = property on="Cell Position" class="DigNum (strict)"("DisabledEnum"=T7."Disabled and Grayed Out" ("Disabled")) -> ()  [unwired: 2 in, 2 out]
      n79 = call "Disable and grey out controls.vi"("Control Label.Text Array"=w85, "error in (no error)"=w84, "VI ref"=w83) -> ()  [unwired: 9 in]
    }
    frame #2 {
      w91 = 0 ("index")
      n80 = call "Load saved scan settings_arbitray cluster elements.vi"() -> ("Scan settings array"=w90:T3[], "Scan settings name array"=w92:string[], "Settings folder path"=w94:path)  [unwired: 8 in, 1 out]
      n81 = property on="Check Saved Settings" class="Ring (strict)"("Strings []"=w92) -> ()  [unwired: 2 in, 2 out]
      n82 = property on="Scan settings in queue" class="Ring (strict)"("Strings []"=w92) -> ()  [unwired: 2 in, 2 out]
      n83 = property on="Save New Settings As..." class="Str"("Value"="") -> ()  [unwired: 2 in, 2 out]
      n84 = Index Array(array=w90, index=w91) -> (element=w93:T3)
      n85 = property on="Check Saved Settings" class="Ring (strict)"("Value"=w91) -> ()  [unwired: 2 in, 2 out]
      n86 = property on="Scan settings" class="Clust (strict)"("Value"=w93) -> (error out=w86:errorcluster)  [unwired: 2 in, 1 out]
      n87 = property class="VI"(error in=w86) -> ("Panel"=w88:refnum<vi>)  [unwired: 1 in, 2 out]
      n88 = property on="Scan settings" class="Clust (strict)"(error in=w86) -> ("Controls[]"=w87:refnum<vi>[])  [unwired: 1 in, 2 out]
    }
    frame #3 {
      # "Import initial scan settings and correct disable/enable logic"
      n89 = local read "J-V cont. Lab.txt array"() -> (w102:string[])
      n90 = local read "J-V cond. cont. Lab.txt array"() -> (w103:string[])
      n91 = property on="No. of scan rate steps" class="DigNum (strict)"() -> ("Value"=w115:dbl)  [unwired: 2 in, 2 out]
      n92 = property on="Scan rate voltage step priority" class="Bool (strict)"() -> ("Value"=w114:bool)  [unwired: 2 in, 2 out]
      n93 = property on="Scan rate measurement delay priority" class="Bool (strict)"() -> ("Value"=w113:bool)  [unwired: 2 in, 2 out]
      n94 = property on="Repeat light scans" class="Bool (strict)"() -> ("Value"=w118:bool)  [unwired: 2 in, 2 out]
      n95 = property on="J-V scan" class="Bool (strict)"() -> ("Value"=w111:bool)  [unwired: 2 in, 2 out]
      n96 = Greater?(x=w115, y=1.0) -> (0:w117:bool)
      n97 = Build Array(w117, w114, w113, w118, w118) -> (w112:bool[])
      n98 = call "Disable-enable scan settgin controls.vi"("VI ref"=w99, "Scan settings control ref array"=w98, "Control Label.Text Array"=w102, "Cond. Control Label.Text Array"=w103, "Cond. Values array"=w112, "Enable?"=w111) -> ("error out"=w100:errorcluster)  [unwired: 9 in]
      n99 = local read "J-t cont. Lab.txt array"() -> (w104:string[])
      n100 = property on="J-t scan" class="Bool (strict)"() -> ("Value"=w110:bool)  [unwired: 2 in, 2 out]
      n101 = call "Disable-enable scan settgin controls.vi"("VI ref"=w99, "Scan settings control ref array"=w98, "Control Label.Text Array"=w104, "error in (no error)"=w100, "Enable?"=w110) -> ("error out"=w101:errorcluster)  [unwired: 10 in]
      n102 = local read "Max P cont. Lab.txt array"() -> (w105:string[])
      n103 = local read "Max P cond. cont. Lab.txt array"() -> (w106:string[])
      n104 = property on="Max P stab. Specific voltage" class="Bool (strict)"() -> ("Value"=w108:bool)  [unwired: 2 in, 2 out]
      n105 = property on="Max. power stabilisation" class="Bool (strict)"() -> ("Value"=w107:bool)  [unwired: 2 in, 2 out]
      n106 = Build Array(w108) -> (w109:bool[])
      n107 = call "Disable-enable scan settgin controls.vi"("VI ref"=w99, "Scan settings control ref array"=w98, "Control Label.Text Array"=w105, "Cond. Control Label.Text Array"=w106, "error in (no error)"=w101, "Cond. Values array"=w109, "Enable?"=w107) -> ()  [unwired: 8 in, 1 out]
    }
  }
  n108 = while {
    shift-right: [w120] -> _
    shift-left: w2 -> [w123]
    tunnel: w3 -> [w122]
    shift-right: [w121] -> _
    shift-left: w1 -> [w124]
    shift-right: [w125] -> _
    shift-left: State_Enumerate_Ring."Initialise" ("Enum") -> [w126]
    stop <- w119 stop-if-true
    n109 = case shown="\"Idle\"" w126 {
      tunnel: [w128 w195 w623 w1140] -> w125
      tunnel: w124 -> [w130 w200 w625 w1142]
      tunnel: w123 -> [w129 w199 w622 w1141]
      tunnel: w122 -> [_ w198 _ _]
      tunnel: [w130 w197 w625 w1142] -> w121
      tunnel: [w129 w196 w622 w1141] -> w120
      tunnel: [FALSE ("Value") w193 FALSE ("Value") FALSE ("Value")] -> w119
      frame "Initialise", Default {
        n110 = stacked-sequence {
          tunnel: [_ _ _ _ _ _ State_Enumerate_Ring."Idle" ("Enum")] -> w128
          frame #0 {
            n111 = call "Login"("Enable"=TRUE) -> ("Manual Mode"=w131:bool, "Experiment Title"=w133:string, "Username"=w134:string)  [unwired: 14 in, 2 out]
            n112 = local write "Experiment Title"(w133) -> ()
            n113 = local write "User Name"(w134) -> ()
            n114 = local write "Manual mode"(w131) -> ()
          }
          frame #1 {
            "Status:" <- "Initialising..." ("Instrument status")
          }
          frame #2 {
            n115 = while {
              stop <- w148 stop-if-true
              n116 = call "Check Keithley is connected.vi"() -> ("error out"=w152:errorcluster)  [unwired: 11 in]
              n117 = Unbundle By Name(w152) -> ("status"=w145:bool)
              n118 = call "Check pcb cont is connected.vi"("error in (no error)"=w152) -> ("error out"=w151:errorcluster)  [unwired: 10 in]
              n119 = Not(x=w145) -> (.not. x?=w144:bool)
              "Keithley 2400" <- w144
              n120 = Unbundle By Name(w151) -> ("status"=w143:bool)
              n121 = call "Check stage contr is connected.vi"("error in (no error)"=w151) -> ("error out"=w139:errorcluster)  [unwired: 10 in]
              n122 = Not(x=w143) -> (.not. x?=w140:bool)
              "PCB controller" <- w140
              n123 = Unbundle By Name(w139) -> ("status"=w142:bool)
              n124 = call "Check Arduino is connected.vi"("Error In"=w139) -> ("error out"=w138:errorcluster)  [unwired: 10 in]
              n125 = Not(x=w142) -> (.not. x?=w141:bool)
              "X-Y stage controller" <- w141
              n126 = Unbundle By Name(w138) -> ("status"=w137:bool)
              n127 = Not(x=w137) -> (.not. x?=w136:bool)
              "Arduino" <- w136
              n128 = Compound Arithmetic op=OR(w144, w140, w141, w136) -> (w149:bool)
              n129 = case shown="False" w149 {
                tunnel: ["Initialising..." ("Instrument status") "Ready!" ("Instrument status")] -> w150
                tunnel: [w153 FALSE ("T button?")] -> w147
                frame False {
                  n130 = Two Button Dialog(message="Something went wrong!\n\nCheck instrument connections.") -> (T button?=w153:bool)  [unwired: 2 in]
                }
                frame True {
                }
              }
              n131 = Not(x=w147) -> (.not. x?=w146:bool)
              n132 = Or(x=w146, y=w149) -> (x .or. y?=w148:bool)
              n133 = local write "Status:"(w150) -> ()
            }
          }
          frame #3 {
            n134 = flat-sequence {
              frame #0 {
                w158 = u16 0 items=["PCB-Keithley", "PCB-EQE", "Manual-Keithley", "Manual-EQE"] ("Experiment type")
                n135 = local write "Status:"("Calibrating filter wheel..." ("Instrument status:")) -> ()
                n136 = call "Set pins on switch board.vi"("Experiment type"=w158) -> ()  [unwired: 10 in, 1 out]
                "Experiment type" <- w158
              }
              frame #1 {
                n137 = call "Move stage to diode position.vi"() -> ("error out"=w161:errorcluster)  [unwired: 11 in]
                n138 = call "Select pin on PCB.vi"("Pin"=128, "error in"=w161) -> ("error out"=w162:errorcluster)  [unwired: 8 in]
                n139 = call "Calibrate filter wheel.vi"("Error In"=w162) -> ("error out"=w163:errorcluster, "Rotation time (ms)"=w164:dbl, "VISA resource name out"=w165:refnum<visa-resource-name>)  [unwired: 6 in, 2 out]
                n140 = call "Find highest intensity filter position.vi"("error in"=w163, "Measurement time (ms)"=w164, "VISA resource name out"=w165) -> ("Angle to no filter (deg.)"=w166:sgl)  [unwired: 7 in, 1 out]
                n141 = call "Turn filter wheel by angle.vi"("Angle (degrees)"=w166) -> ("Enable Channel out"=w168:u8, "Serial Port out"=w167:refnum<visa-resource-name>)  [unwired: 8 in, 1 out]
                n142 = call "Disable Motor.vi"("Enable Channel"=w168, "Serial Port"=w167) -> ()  [unwired: 9 in, 1 out]
              }
              frame #2 {
                n143 = local write "Status:"("Ready!" ("Instrument status:")) -> ()
                "Current Angle (degrees)" <- 0.0 ("Current Angle (degrees)")
              }
            }
          }
          frame #4 {
            n144 = property on="Manual mode" class="Bool (strict)"() -> ("Value"=w171:bool)  [unwired: 2 in, 2 out]
            n145 = case shown="True" w171 {
              frame False {
                # "Move to 0,0 to reset stage co-ordinates,\nthen to load position"
                n146 = One Button Dialog(message="The stage is about to move\nto the sample loading position.\n\nAre you ready?") -> (true=w173:bool)  [unwired: 1 in]
                n147 = Not(x=w173) -> (.not. x?=w172:bool)
                n148 = Bundle By Name(cluster=errorcluster {"status"=FALSE, "code"=0, "source"=""} ("error in (no error) 3"), "status"=w172) -> (w174:errorcluster)
                n149 = call "Move X-Y to L-.vi"("error in (no error) 3"=w174) -> ("error out 3"=w177:errorcluster)  [unwired: 7 in, 3 out]
                n150 = Concatenate Strings("X", "10000") -> (w181:string)
                n151 = Concatenate Strings("Y", "20000") -> (w180:string)
                n152 = call "Move X-Y to specific position.vi"("error in (no error) 3"=w177, "position 2"=w180, "position 1"=w181) -> ()  [unwired: 4 in, 5 out]
              }
              frame True {
                w184 = u16 2 items=["PCB-Keithley", "PCB-EQE", "Manual-Keithley", "Manual-EQE"] ("Experiment type")
                n153 = call "Set pins on switch board.vi"("Experiment type"=w184) -> ()  [unwired: 10 in, 1 out]
                n154 = local write "Experiment type"(w184) -> ()
              }
            }
          }
          frame #5 {
            n155 = local write "Status:"("Ready!" ("Status:")) -> ()
            n156 = One Button Dialog(message="The system is ready.\n\nYou may now setup the experiment.") -> ()  [unwired: 1 in, 1 out]
          }
          frame #6 {
            n157 = local read "User Name"() -> (w188:string)
            n158 = Equal?(x=w188, y="James B") -> (x = y?=w187:bool)
            n159 = case shown="True" w187 {
              frame False {
                n160 = property on="Set diode pos" class="Bool (strict)"("DisabledEnum"=T7."Disabled and Grayed Out" ("Disabled")) -> ()  [unwired: 2 in, 2 out]
              }
              frame True {
                n161 = property on="Set diode pos" class="Bool (strict)"("DisabledEnum"=T7."Enabled" ("Disabled")) -> ()  [unwired: 2 in, 2 out]
              }
            }
          }
        }
      }
      frame "Idle" {
        n162 = property on="Exit Program" class="Bool (strict)"("DisabledEnum"=T7."Enabled" ("Disabled")) -> ()  [unwired: 2 in, 2 out]
        n163 = event shown="[19] \"Save new settings\": Mouse Down" {
          selector: _ -> [_ _ _ _ _ _ _ _ _ _ _ _ _ _ _ _ _ _ _ _ _ _ _ _ _ _ _ _ _ _ _ _ _]
          dyn-events: _ -> [_ _ _ _ _ _ _ _ _ _ _ _ _ _ _ _ _ _ _ _ _ _ _ _ _ _ _ _ _ _ _ _ _]
          timeout: _ -> [_ _ _ _ _ _ _ _ _ _ _ _ _ _ _ _ _ _ _ _ _ _ _ _ _ _ _ _ _ _ _ _ _]
          tunnel: 0 -> [w211 _ w231 _ w251 _ w271 _ w294 w303 _ _ _ _ _ _ _ _ _ _ _ _ _ _ _ _ _ _ _ _ _ _ _]
          tunnel: "error in (no error) 3" -> [w210 _ w230 _ w250 _ w270 _ w293 w302 _ _ _ _ _ _ _ _ _ _ _ _ _ _ _ _ _ _ _ _ _ _ _]
          tunnel: w200 -> [w205 w215 w225 w235 w245 w255 w265 w275 w285 w298 w319 w325 w330 w340 w350 w357 w367 w372 w382 w393 w413 w425 w484 w525 w535 w547 w555 w566 w577 w588 w600 w609 w620]
          tunnel: w199 -> [w204 w214 w224 w234 w244 w254 w264 w274 w284 w297 w318 w324 w329 w339 w349 w356 w366 w371 w381 w392 w412 w426 w489 w524 w534 w546 w554 w565 w576 w587 w599 w608 w619]
          tunnel: w198 -> [_ _ _ _ _ _ _ _ _ _ _ _ _ _ _ _ _ _ _ w397 w414 w422 _ _ _ _ _ _ _ _ _ _ _]
          tunnel: [w205 w215 w225 w235 w245 w255 w265 w275 w285 w298 w319 w325 w330 w340 w350 w357 w367 w372 w382 w396 w413 w424 w482 w525 w535 w547 w555 w566 w577 w588 w600 w609 w620] -> w197
          tunnel: [w204 w214 w224 w234 w244 w254 w264 w274 w284 w297 w318 w324 w329 w339 w349 w356 w366 w371 w381 w395 w412 w423 w480 w524 w534 w546 w554 w565 w576 w587 w599 w608 w619] -> w196
          tunnel: [State_Enumerate_Ring."Idle" ("Enum") State_Enumerate_Ring."Idle" ("Enum") State_Enumerate_Ring."Idle" ("Enum") State_Enumerate_Ring."Idle" ("Enum") State_Enumerate_Ring."Idle" ("Enum") State_Enumerate_Ring."Idle" ("Enum") State_Enumerate_Ring."Idle" ("Enum") State_Enumerate_Ring."Idle" ("Enum") State_Enumerate_Ring."Idle" ("Enum") State_Enumerate_Ring."Idle" ("Enum") State_Enumerate_Ring."Idle" ("Enum") State_Enumerate_Ring."Idle" ("Enum") State_Enumerate_Ring."Idle" ("Enum") State_Enumerate_Ring."Idle" ("Enum") State_Enumerate_Ring."Idle" ("Enum") State_Enumerate_Ring."Idle" ("Enum") State_Enumerate_Ring."Idle" ("Enum") State_Enumerate_Ring."Idle" ("Enum") State_Enumerate_Ring."Idle" ("Enum") State_Enumerate_Ring."Idle" ("Enum") State_Enumerate_Ring."Idle" ("Enum") State_Enumerate_Ring."Idle" ("Enum") State_Enumerate_Ring."Idle" ("Enum") State_Enumerate_Ring."Idle" ("Enum") State_Enumerate_Ring."Measure" ("Enum") State_Enumerate_Ring."Idle" ("Enum") State_Enumerate_Ring."Idle" ("Enum") State_Enumerate_Ring."Idle" ("Enum") State_Enumerate_Ring."Idle" ("Enum") State_Enumerate_Ring."Idle" ("Enum") State_Enumerate_Ring."Idle" ("Enum") State_Enumerate_Ring."Idle" ("Enum") State_Enumerate_Ring."Idle" ("Enum")] -> w195
          tunnel: [FALSE ("Value") FALSE ("Value") FALSE ("Value") FALSE ("Value") FALSE ("Value") FALSE ("Value") FALSE ("Value") FALSE ("Value") FALSE ("Value") FALSE ("Value") FALSE ("Value") FALSE ("Value") FALSE ("Value") FALSE ("Value") FALSE ("Value") FALSE ("Value") FALSE ("Value") FALSE ("Value") FALSE ("Value") FALSE ("Value") FALSE ("Value") FALSE ("Value") w479 FALSE ("Value") FALSE ("Value") FALSE ("Value") FALSE ("Value") FALSE ("Value") FALSE ("Value") FALSE ("Value") FALSE ("Value") FALSE ("Value") w617] -> w193
          event "X +ve": Mouse Down {
            n164 = event-data() -> ()  [unwired: 1 in, 1 out]
            n165 = call "Enable stage.vi"("error in (no error)"=w210, "Ref in"=w211) -> ("error out"=w208:errorcluster, "reference (out)"=w209:i32)  [unwired: 8 in]
            n166 = call "sendReceiveCommand.vi"("reference (in)"=w209, "write_string"="JX+" ("raw_cmd"), "error in (no error)"=w208) -> ("reference (out)"=→"reference (out)":i32)  [unwired: 10 in, 2 out]
          }
          event "X +ve": Mouse Up {
            n167 = event-data() -> ()  [unwired: 1 in, 1 out]
            n168 = local read "reference (out)"() -> (w221:i32)
            n169 = call "sendReceiveCommand.vi"("reference (in)"=w221, "write_string"="ABORT" ("raw_cmd")) -> ("reference (out)"=w220:i32, "error out"=w219:errorcluster)  [unwired: 11 in, 1 out]
            n170 = call "Disable stage.vi"("error in (no error)"=w219, "reference (out)"=w220) -> ("X Pos"=w217:string, "Y Pos"=w218:string)  [unwired: 8 in]
            n171 = local write "Y position"(w218) -> ()
            n172 = local write "X position"(w217) -> ()
          }
          event "X -ve": Mouse Down {
            n173 = event-data() -> ()  [unwired: 1 in, 1 out]
            n174 = call "Enable stage.vi"("error in (no error)"=w230, "Ref in"=w231) -> ("error out"=w228:errorcluster, "reference (out)"=w229:i32)  [unwired: 8 in]
            n175 = call "sendReceiveCommand.vi"("reference (in)"=w229, "write_string"="JX-" ("raw_cmd"), "error in (no error)"=w228) -> ("reference (out)"=→"reference (out) 2":i32)  [unwired: 10 in, 2 out]
          }
          event "X -ve": Mouse Up {
            n176 = event-data() -> ()  [unwired: 1 in, 1 out]
            n177 = local read "reference (out) 2"() -> (w241:i32)
            n178 = call "sendReceiveCommand.vi"("reference (in)"=w241, "write_string"="ABORT" ("raw_cmd")) -> ("reference (out)"=w240:i32, "error out"=w239:errorcluster)  [unwired: 11 in, 1 out]
            n179 = call "Disable stage.vi"("error in (no error)"=w239, "reference (out)"=w240) -> ("X Pos"=w237:string, "Y Pos"=w238:string)  [unwired: 8 in]
            n180 = local write "Y position"(w238) -> ()
            n181 = local write "X position"(w237) -> ()
          }
          event "Y +ve": Mouse Down {
            n182 = event-data() -> ()  [unwired: 1 in, 1 out]
            n183 = call "Enable stage.vi"("error in (no error)"=w250, "Ref in"=w251) -> ("error out"=w248:errorcluster, "reference (out)"=w249:i32)  [unwired: 8 in]
            n184 = call "sendReceiveCommand.vi"("reference (in)"=w249, "write_string"="JY+" ("raw_cmd"), "error in (no error)"=w248) -> ("reference (out)"=→"reference (out) 3":i32)  [unwired: 10 in, 2 out]
          }
          event "Y +ve": Mouse Up {
            n185 = event-data() -> ()  [unwired: 1 in, 1 out]
            n186 = local read "reference (out) 3"() -> (w261:i32)
            n187 = call "sendReceiveCommand.vi"("reference (in)"=w261, "write_string"="ABORT" ("raw_cmd")) -> ("reference (out)"=w260:i32, "error out"=w259:errorcluster)  [unwired: 11 in, 1 out]
            n188 = call "Disable stage.vi"("error in (no error)"=w259, "reference (out)"=w260) -> ("X Pos"=w257:string, "Y Pos"=w258:string)  [unwired: 8 in]
            n189 = local write "X position"(w257) -> ()
            n190 = local write "Y position"(w258) -> ()
          }
          event "Y -ve": Mouse Down {
            n191 = event-data() -> ()  [unwired: 1 in, 1 out]
            n192 = call "Enable stage.vi"("error in (no error)"=w270, "Ref in"=w271) -> ("error out"=w268:errorcluster, "reference (out)"=w269:i32)  [unwired: 8 in]
            n193 = call "sendReceiveCommand.vi"("reference (in)"=w269, "write_string"="JY-" ("raw_cmd"), "error in (no error)"=w268) -> ("reference (out)"=→"reference (out) 4":i32)  [unwired: 10 in, 2 out]
          }
          event "Y -ve": Mouse Up {
            n194 = event-data() -> ()  [unwired: 1 in, 1 out]
            n195 = local read "reference (out) 4"() -> (w281:i32)
            n196 = call "sendReceiveCommand.vi"("reference (in)"=w281, "write_string"="ABORT" ("raw_cmd")) -> ("reference (out)"=w280:i32, "error out"=w279:errorcluster)  [unwired: 11 in, 1 out]
            n197 = call "Disable stage.vi"("error in (no error)"=w279, "reference (out)"=w280) -> ("X Pos"=w277:string, "Y Pos"=w278:string)  [unwired: 8 in]
            n198 = local write "Y position"(w278) -> ()
            n199 = local write "X position"(w277) -> ()
          }
          event "Go to negative limit": Mouse Down {
            n200 = event-data() -> ()  [unwired: 1 in, 1 out]
            n201 = call "Enable stage.vi"("error in (no error)"=w293, "Ref in"=w294) -> ("error out"=w291:errorcluster, "reference (out)"=w292:i32)  [unwired: 8 in]
            n202 = call "sendReceiveCommand.vi"("reference (in)"=w292, "write_string"="L-" ("raw_cmd"), "error in (no error)"=w291) -> ("reference (out)"=w290:i32, "error out"=w289:errorcluster)  [unwired: 10 in, 1 out]
            n203 = call "Disable stage.vi"("error in (no error)"=w289, "reference (out)"=w290) -> ("X Pos"=w287:string, "Y Pos"=w288:string)  [unwired: 8 in]
            n204 = local write "Y position"(w288) -> ()
            n205 = local write "X position"(w287) -> ()
          }
          event "Set diode pos": Mouse Down {
            n206 = event-data() -> ()  [unwired: 1 in, 1 out]
            n207 = call "Enable stage.vi"("error in (no error)"=w302, "Ref in"=w303) -> ("error out"=w300:errorcluster, "reference (out)"=w301:i32)  [unwired: 8 in]
            n208 = call "sendReceiveCommand.vi"("reference (in)"=w301, "write_string"="PX" ("raw_cmd"), "error in (no error)"=w300) -> ("reference (out)"=w315:i32, "read_string"=w312:string, "error out"=w314:errorcluster)  [unwired: 10 in]
            n209 = call "sendReceiveCommand.vi"("reference (in)"=w315, "write_string"="PY" ("raw_cmd"), "error in (no error)"=w314) -> ("reference (out)"=w307:i32, "read_string"=w311:string, "error out"=w306:errorcluster)  [unwired: 10 in]
            n210 = Build Array(w312, w311) -> (w310:string[])
            n211 = call-poly <vilib>:"Write To Spreadsheet File.vi"("append to file? (new file:F)"=FALSE, "1D data"=w310, "file path (dialog if empty)"=path "C:/Automated SS files/DiodeXY.txt") -> ()  [unwired: 5 in, 1 out]
            n212 = call "Disable stage.vi"("error in (no error)"=w306, "reference (out)"=w307) -> ("X Pos"=→"X position":string, "Y Pos"=→"Y position":string)  [unwired: 8 in]
          }
          event "Load details from file": Mouse Down {
            n213 = event-data() -> ()  [unwired: 1 in, 1 out]
            n214 = call "Upload info from spreadsheet.vi"() -> ("Cell Settings Array 1"=w321:T2)  [unwired: 11 in]
            n215 = local write "Cell Settings Array 1"(w321) -> ()
          }
          event "Save details to file": Mouse Down {
            n216 = event-data() -> ()  [unwired: 1 in, 1 out]
            n217 = local read "Cell Settings Array 1"() -> (w323:T2)
            n218 = call "Save info to spreadsheet.vi"("Cell Settings Array"=w323) -> ()  [unwired: 11 in]
          }
          event Value Change {
            n219 = event-data() -> ()  [unwired: 1 in, 5 out]
            n220 = property on="Max power tracking" class="Bool (strict)"() -> ("Value"=w331:bool)  [unwired: 2 in, 2 out]
            n221 = case shown="False" w331 {
              frame False {
                n222 = property on="Max P stab. Specific voltage" class="Bool (strict)"() -> ("Value"=w332:bool)  [unwired: 2 in, 2 out]
                n223 = case shown="False" w332 {
                  frame False {
                    n224 = property on="Vmp (V)" class="DigNum (strict)"("DisabledEnum"=T7."Disabled and Grayed Out" ("Disabled")) -> ()  [unwired: 2 in, 2 out]
                  }
                  frame True {
                    n225 = property on="Vmp (V)" class="DigNum (strict)"("DisabledEnum"=T7."Enabled" ("Disabled")) -> ()  [unwired: 2 in, 2 out]
                  }
                }
              }
              frame True {
                w335 = FALSE ("Value")
                n226 = property on="Vmp from J-V scan" class="Bool (strict)"("Value"=w335) -> ()  [unwired: 2 in, 2 out]
                n227 = property on="Max P stab. Specific voltage" class="Bool (strict)"("Value"=w335) -> ()  [unwired: 2 in, 2 out]
                n228 = property on="Vmp (V)" class="DigNum (strict)"("DisabledEnum"=T7."Disabled and Grayed Out" ("Disabled")) -> ()  [unwired: 2 in, 2 out]
              }
            }
          }
          event Value Change {
            n229 = event-data() -> ()  [unwired: 1 in, 5 out]
            n230 = property on="Vmp from J-V scan" class="Bool (strict)"() -> ("Value"=w341:bool)  [unwired: 2 in, 2 out]
            n231 = case shown="False" w341 {
              frame False {
                n232 = property on="Max P stab. Specific voltage" class="Bool (strict)"() -> ("Value"=w342:bool)  [unwired: 2 in, 2 out]
                n233 = case shown="False" w342 {
                  frame False {
                    n234 = property on="Vmp (V)" class="DigNum (strict)"("DisabledEnum"=T7."Disabled and Grayed Out" ("Disabled")) -> ()  [unwired: 2 in, 2 out]
                  }
                  frame True {
                    n235 = property on="Vmp (V)" class="DigNum (strict)"("DisabledEnum"=T7."Enabled" ("Disabled")) -> ()  [unwired: 2 in, 2 out]
                  }
                }
              }
              frame True {
                w346 = FALSE ("Value")
                n236 = property on="Max P stab. Specific voltage" class="Bool (strict)"("Value"=w346) -> ()  [unwired: 2 in, 2 out]
                n237 = property on="Vmp (V)" class="DigNum (strict)"("DisabledEnum"=T7."Disabled and Grayed Out" ("Disabled")) -> ()  [unwired: 2 in, 2 out]
                n238 = property on="Max power tracking" class="Bool (strict)"("Value"=w346) -> ()  [unwired: 2 in, 2 out]
              }
            }
          }
          event Value Change {
            n239 = event-data() -> ()  [unwired: 1 in, 5 out]
            n240 = property on="Max P stab. Specific voltage" class="Bool (strict)"() -> ("Value"=w351:bool)  [unwired: 2 in, 2 out]
            n241 = case shown="False" w351 {
              frame False {
                n242 = property on="Vmp (V)" class="DigNum (strict)"("DisabledEnum"=T7."Disabled and Grayed Out" ("Disabled")) -> ()  [unwired: 2 in, 2 out]
              }
              frame True {
                w354 = FALSE ("Value")
                n243 = property on="Vmp from J-V scan" class="Bool (strict)"("Value"=w354) -> ()  [unwired: 2 in, 2 out]
                n244 = property on="Max power tracking" class="Bool (strict)"("Value"=w354) -> ()  [unwired: 2 in, 2 out]
                n245 = property on="Vmp (V)" class="DigNum (strict)"("DisabledEnum"=T7."Enabled" ("Disabled")) -> ()  [unwired: 2 in, 2 out]
              }
            }
          }
          event "Change pin on pcb": Mouse Down {
            n246 = event-data() -> ()  [unwired: 1 in, 1 out]
            n247 = Decrement(x="Cell") -> (x-1=w363:i64)
            n248 = Multiply(x=8, y=w363) -> (x*y=w361:i64)
            n249 = Add(x=w361, y="Pixel") -> (x+y=w359:i64)
            "Pin" <- w359
            n250 = call "Select pin on PCB.vi"("Pin"=w359) -> ()  [unwired: 9 in, 1 out]
          }
          event "Measure current": Mouse Down {
            n251 = event-data() -> ()  [unwired: 1 in, 1 out]
            n252 = call "Measure current now.vi"() -> ("Current"=→"Current (A)":dbl)  [unwired: 11 in]
          }
          event "Shutter open": Mouse Down {
            n253 = event-data() -> ()  [unwired: 1 in, 1 out]
            n254 = call <instrlib>:"Initialize.vi"("VISA resource name"=refnum<visa-resource-name> "GPIB0::24::INSTR") -> ("error out"=w379:errorcluster, "VISA resource name out"=w378:refnum<visa-resource-name>)  [unwired: 4 in, 5 out]
            n255 = call <instrlib>:"Set IO Pins.vi"("error in (no error)"=w379, "Output Pattern (0)"=0 ("Numeric"), "VISA resource name"=w378) -> ("error out"=w376:errorcluster, "VISA resource name out"=w375:refnum<visa-resource-name>)  [unwired: 7 in]
            n256 = call <instrlib>:"Close.vi"("error in (no error)"=w376, "VISA resource name"=w375) -> ()  [unwired: 9 in, 1 out]
          }
          event "Shutter closed": Mouse Down {
            n257 = event-data() -> ()  [unwired: 1 in, 1 out]
            n258 = call <instrlib>:"Initialize.vi"("VISA resource name"=refnum<visa-resource-name> "GPIB0::24::INSTR") -> ("error out"=w389:errorcluster, "VISA resource name out"=w388:refnum<visa-resource-name>)  [unwired: 4 in, 5 out]
            n259 = call <instrlib>:"Set IO Pins.vi"("error in (no error)"=w389, "Output Pattern (0)"=1 ("Numeric"), "VISA resource name"=w388) -> ("error out"=w386:errorcluster, "VISA resource name out"=w385:refnum<visa-resource-name>)  [unwired: 7 in]
            n260 = call <instrlib>:"Close.vi"("error in (no error)"=w386, "VISA resource name"=w385) -> ()  [unwired: 9 in, 1 out]
          }
          event "Save new settings": Mouse Down {
            n261 = event-data() -> ()  [unwired: 1 in, 7 out]
            n262 = Not Equal?(x="Save New Settings As...", y="") -> (x != y?=w390:bool)
            n263 = case shown="True" w390 {
              tunnel: [w400 w407] -> w395
              tunnel: [w401 w406] -> w396
              tunnel: w397 -> [_ w409]
              tunnel: "Save New Settings As..." -> [_ w405]
              tunnel: w393 -> [w401 _]
              tunnel: w392 -> [w400 _]
              frame False {
              }
              frame True {
                n264 = call "Save scan settings.vi"("Path"=w409, "New scan settings"="Scan settings", "New name"=w405) -> ("error out"=w402:errorcluster)  [unwired: 8 in]
                n265 = call "Load saved scan settings_arbitray cluster elements.vi"("error in (no error)"=w402) -> ("Scan settings array"=w407:T3[], "Scan settings name array"=w406:string[])  [unwired: 7 in, 2 out]
                n266 = Search 1D Array(1D array=w406, element=w405) -> (index of element=w404:i32)  [unwired: 1 in]
                n267 = property on="Check Saved Settings" class="Ring (strict)"("Strings []"=w406) -> ()  [unwired: 2 in, 2 out]
                n268 = property on="Check Saved Settings" class="Ring (strict)"("Value"=w404) -> ()  [unwired: 2 in, 2 out]
                n269 = property on="Save New Settings As..." class="Str"(error in=w402, "Value"="") -> ()  [unwired: 1 in, 2 out]
                n270 = property on="Scan settings in queue" class="Ring (strict)"("Strings []"=w406) -> ()  [unwired: 2 in, 2 out]
              }
            }
          }
          event "Update": Mouse Down {
            n271 = event-data() -> ()  [unwired: 1 in, 7 out]
            n272 = property on="Check Saved Settings" class="Ring (strict)"() -> ("Strings []"=w418:string[])  [unwired: 2 in, 2 out]
            n273 = property on="Check Saved Settings" class="Ring (strict)"() -> ("Value"=w417:u16)  [unwired: 2 in, 2 out]
            n274 = local read "Scan settings"() -> (w415:T3)
            n275 = Index Array(array=w418, index=w417) -> (element=w416:string)
            n276 = call "Save scan settings.vi"("Path"=w414, "New scan settings"=w415, "New name"=w416) -> ()  [unwired: 8 in, 1 out]
          }
          event "Delete settings": Mouse Down {
            n277 = event-data() -> ()  [unwired: 1 in, 7 out]
            n278 = property on="Delete settings" class="Bool (strict)"() -> ("Value"=w421:bool)  [unwired: 2 in, 2 out]
            n279 = case shown="True" w421 {
              tunnel: w426 -> [w427 w434]
              tunnel: w425 -> [w428 w433]
              tunnel: [w428 w432] -> w424
              tunnel: [w427 w431] -> w423
              tunnel: w422 -> [_ w430]
              frame False {
              }
              frame True {
                n280 = property on="Check Saved Settings" class="Ring (strict)"() -> ("Strings []"=w440:string[])  [unwired: 2 in, 2 out]
                n281 = property on="Check Saved Settings" class="Ring (strict)"() -> ("Value"=w439:u16)  [unwired: 2 in, 2 out]
                n282 = Index Array(array=w440, index=w439) -> (element=w429:string)
                n283 = Concatenate Strings("Are you sure you want to delete " ("string"), w429, "?" ("string")) -> (w436:string)
                n284 = Two Button Dialog(message=w436, 1:"No" ("F button name (\"Cancel\")"), 2:"Yes" ("T button name (\"OK\")")) -> (T button?=w435:bool)
                n285 = case shown="True" w435 {
                  tunnel: w434 -> [w443 _]
                  tunnel: w433 -> [w444 _]
                  tunnel: [w444 w450] -> w432
                  tunnel: [w443 w449] -> w431
                  tunnel: w430 -> [_ w456]
                  tunnel: w429 -> [_ w455]
                  frame False {
                  }
                  frame True {
                    w453 = 0 ("index")
                    n286 = call "Delete scan settings.vi"("Path"=w456, "Scan settings name"=w455) -> ("error out"=w448:errorcluster)  [unwired: 9 in]
                    n287 = call "Load saved scan settings_arbitray cluster elements.vi"("error in (no error)"=w448) -> ("Scan settings array"=w449:T3[], "Scan settings name array"=w450:string[])  [unwired: 7 in, 2 out]
                    n288 = property on="Scan settings in queue" class="Ring (strict)"("Strings []"=w450) -> (error out=w451:errorcluster)  [unwired: 2 in, 1 out]
                    n289 = property on="Check Saved Settings" class="Ring (strict)"(error in=w451, "Strings []"=w450) -> (error out=w452:errorcluster)  [unwired: 1 in, 1 out]
                    n290 = Index Array(array=w449, index=w453) -> (element=w454:T3)
                    n291 = property on="Check Saved Settings" class="Ring (strict)"(error in=w452, "Value"=w453) -> ()  [unwired: 1 in, 2 out]
                    n292 = property on="Scan settings" class="Clust (strict)"(error in=w452, "Value"=w454) -> (error out=w447:errorcluster)  [unwired: 1 in, 1 out]
                    n293 = flat-sequence {
                      tunnel: w447 -> [w459]
                      tunnel: [w458] -> w446
                      tunnel: [w457] -> w445
                      tunnel: w446 -> [w476]
                      tunnel: w445 -> [w475]
                      frame #0 {
                        n294 = property class="VI"(error in=w459) -> ("Panel"=w458:refnum<vi>)  [unwired: 1 in, 2 out]
                        n295 = property on="Scan settings" class="Clust (strict)"(error in=w459) -> ("Controls[]"=w457:refnum<vi>[])  [unwired: 1 in, 2 out]
                      }
                      frame #1 {
                        n296 = property on="Scan rate voltage step priority" class="Bool (strict)"() -> ("Value"=w470:bool)  [unwired: 2 in, 2 out]
                        n297 = property on="Scan rate measurement delay priority" class="Bool (strict)"() -> ("Value"=w469:bool)  [unwired: 2 in, 2 out]
                        n298 = property on="Repeat light scans" class="Bool (strict)"() -> ("Value"=w468:bool)  [unwired: 2 in, 2 out]
                        n299 = property on="J-V cond. cont. Lab.txt array" class="Arr (strict)"() -> ("Value"=w473:string[])  [unwired: 2 in, 2 out]
                        n300 = property on="J-V cont. Lab.txt array" class="Arr (strict)"() -> ("Value"=w474:string[])  [unwired: 2 in, 2 out]
                        n301 = property on="No. of scan rate steps" class="DigNum (strict)"() -> ("Value"=w477:dbl)  [unwired: 2 in, 2 out]
                        n302 = Greater?(x=w477, y=1.0) -> (0:w471:bool)
                        n303 = property on="J-V scan" class="Bool (strict)"() -> ("Value"=w467:bool)  [unwired: 2 in, 2 out]
                        n304 = Build Array(w471, w470, w469, w468, w468) -> (w472:bool[])
                        n305 = call "Disable-enable scan settgin controls.vi"("VI ref"=w476, "Scan settings control ref array"=w475, "Control Label.Text Array"=w474, "Cond. Control Label.Text Array"=w473, "Cond. Values array"=w472, "Enable?"=w467) -> ()  [unwired: 9 in, 1 out]
                        n306 = property on="J-t cont. Lab.txt array" class="Arr (strict)"() -> ("Value"=w466:string[])  [unwired: 2 in, 2 out]
                        n307 = property on="J-t scan" class="Bool (strict)"() -> ("Value"=w465:bool)  [unwired: 2 in, 2 out]
                        n308 = call "Disable-enable scan settgin controls.vi"("VI ref"=w476, "Scan settings control ref array"=w475, "Control Label.Text Array"=w466, "Enable?"=w465) -> ()  [unwired: 11 in, 1 out]
                        n309 = property on="Max P cont. Lab.txt array" class="Arr (strict)"() -> ("Value"=w464:string[])  [unwired: 2 in, 2 out]
                        n310 = property on="Max P cond. cont. Lab.txt array" class="Arr (strict)"() -> ("Value"=w463:string[])  [unwired: 2 in, 2 out]
                        n311 = property on="Max P stab. Specific voltage" class="Bool (strict)"() -> ("Value"=w461:bool)  [unwired: 2 in, 2 out]
                        n312 = property on="Max. power stabilisation" class="Bool (strict)"() -> ("Value"=w462:bool)  [unwired: 2 in, 2 out]
                        n313 = Build Array(w461) -> (w460:bool[])
                        n314 = call "Disable-enable scan settgin controls.vi"("VI ref"=w476, "Scan settings control ref array"=w475, "Control Label.Text Array"=w464, "Cond. Control Label.Text Array"=w463, "Cond. Values array"=w460, "Enable?"=w462) -> ()  [unwired: 9 in, 1 out]
                      }
                    }
                  }
                }
              }
            }
          }
          event "Check Saved Settings": Value Change {
            n315 = event-data() -> ()  [unwired: 1 in, 1 out]
            n316 = flat-sequence {
              tunnel: w489 -> [w490]
              tunnel: [w494] -> w487
              tunnel: [w493] -> w486
              tunnel: [w492] -> w485
              tunnel: w484 -> [w491]
              tunnel: [w491] -> w483
              tunnel: [w490] -> w481
              tunnel: w487 -> [w500]
              tunnel: w486 -> [w499]
              tunnel: w485 -> [w498]
              tunnel: w483 -> [w502]
              tunnel: [w502] -> w482
              tunnel: w481 -> [w501]
              tunnel: [w501] -> w480
              tunnel: [FALSE ("Value")] -> w479
              frame #0 {
                n317 = Index Array(array=w490, index="Check Saved Settings") -> (element=w495:T3)
                n318 = property on="Scan settings" class="Clust (strict)"("Value"=w495) -> (error out=w492:errorcluster)  [unwired: 2 in, 1 out]
                n319 = property class="VI"(error in=w492) -> ("Panel"=w494:refnum<vi>)  [unwired: 1 in, 2 out]
                n320 = property on="Scan settings" class="Clust (strict)"(error in=w492) -> ("Controls[]"=w493:refnum<vi>[])  [unwired: 1 in, 2 out]
              }
              frame #1 {
                n321 = property on="No. of scan rate steps" class="DigNum (strict)"() -> ("Value"=w512:dbl)  [unwired: 2 in, 2 out]
                n322 = Greater?(x=w512, y=1.0) -> (0:w514:bool)
                n323 = property on="Scan rate voltage step priority" class="Bool (strict)"() -> ("Value"=w511:bool)  [unwired: 2 in, 2 out]
                n324 = property on="Scan rate measurement delay priority" class="Bool (strict)"() -> ("Value"=w510:bool)  [unwired: 2 in, 2 out]
                n325 = property on="Repeat light scans" class="Bool (strict)"() -> ("Value"=w509:bool)  [unwired: 2 in, 2 out]
                n326 = property on="J-V cont. Lab.txt array" class="Arr (strict)"(error in=w498) -> ("Value"=w515:string[])  [unwired: 1 in, 2 out]
                n327 = property on="J-V cond. cont. Lab.txt array" class="Arr (strict)"(error in=w498) -> (error out=w518:errorcluster, "Value"=w516:string[])  [unwired: 1 in, 1 out]
                n328 = property on="J-V scan" class="Bool (strict)"() -> ("Value"=w508:bool)  [unwired: 2 in, 2 out]
                n329 = Build Array(w514, w511, w510, w509, w509) -> (w503:bool[])
                n330 = call "Disable-enable scan settgin controls.vi"("VI ref"=w500, "Scan settings control ref array"=w499, "Control Label.Text Array"=w515, "Cond. Control Label.Text Array"=w516, "Cond. Values array"=w503, "Enable?"=w508) -> ()  [unwired: 9 in, 1 out]
                n331 = property on="J-t cont. Lab.txt array" class="Arr (strict)"(error in=w518) -> (error out=w519:errorcluster, "Value"=w517:string[])  [unwired: 1 in, 1 out]
                n332 = property on="J-t scan" class="Bool (strict)"() -> ("Value"=w505:bool)  [unwired: 2 in, 2 out]
                n333 = call "Disable-enable scan settgin controls.vi"("VI ref"=w500, "Scan settings control ref array"=w499, "Control Label.Text Array"=w517, "Enable?"=w505) -> ()  [unwired: 11 in, 1 out]
                n334 = property on="Max P cont. Lab.txt array" class="Arr (strict)"(error in=w519) -> ("Value"=w520:string[])  [unwired: 1 in, 2 out]
                n335 = property on="Max P cond. cont. Lab.txt array" class="Arr (strict)"(error in=w519) -> ("Value"=w521:string[])  [unwired: 1 in, 2 out]
                n336 = property on="Max. power stabilisation" class="Bool (strict)"() -> ("Value"=w507:bool)  [unwired: 2 in, 2 out]
                n337 = property on="Max P stab. Specific voltage" class="Bool (strict)"() -> ("Value"=w506:bool)  [unwired: 2 in, 2 out]
                n338 = Build Array(w506) -> (w504:bool[])
                n339 = call "Disable-enable scan settgin controls.vi"("VI ref"=w500, "Scan settings control ref array"=w499, "Control Label.Text Array"=w520, "Cond. Control Label.Text Array"=w521, "Cond. Values array"=w504, "Enable?"=w507) -> ()  [unwired: 9 in, 1 out]
              }
            }
          }
          event "Move to load pos.": Mouse Down {
            # "Move to load position"
            n340 = event-data() -> ()  [unwired: 1 in, 7 out]
            n341 = Concatenate Strings("X", "10000") -> (w529:string)
            n342 = Concatenate Strings("Y", "20000") -> (w528:string)
            n343 = call "Move X-Y to specific position.vi"("position 2"=w528, "position 1"=w529) -> ()  [unwired: 5 in, 5 out]
          }
          event "Start Scan": Mouse Down {
            n344 = event-data() -> ()  [unwired: 1 in, 1 out]
            n345 = local read "Scan set. Lab.txt array"() -> (w540:string[])
            n346 = local read "Sample set. Lab.txt array"() -> (w539:string[])
            n347 = local read "Measure Lab.txt array"() -> (w538:string[])
            n348 = local read "Advanced Lab.txt array"() -> (w537:string[])
            n349 = Build Array (concatenate)(w540, w539, w538, w537) -> (w536:string[])
            n350 = property class="VI"() -> (error out=w541:errorcluster, "Panel"=w542:refnum<vi>)  [unwired: 2 in, 1 out]
            n351 = call "Disable and grey out controls.vi"("Control Label.Text Array"=w536, "error in (no error)"=w541, "VI ref"=w542) -> ()  [unwired: 9 in]
            n352 = local write "Status:"("Measuring" ("Status:")) -> ()
          }
          event Value Change {
            n353 = event-data() -> ()  [unwired: 1 in, 5 out]
            n354 = property on="No. of scan rate steps" class="DigNum (strict)"() -> ("Value"=w550:dbl)  [unwired: 2 in, 2 out]
            n355 = Greater?(x=w550, y=1.0) -> (0:w548:bool)
            n356 = case shown="True" w548 {
              frame False {
                n357 = property on="Scan rate max (V/s)" class="DigNum (strict)"("DisabledEnum"=T7."Disabled and Grayed Out" ("Disabled")) -> ()  [unwired: 2 in, 2 out]
              }
              frame True {
                n358 = property on="Scan rate max (V/s)" class="DigNum (strict)"("DisabledEnum"=T7."Enabled" ("Disabled")) -> ()  [unwired: 2 in, 2 out]
              }
            }
          }
          event Value Change {
            n359 = event-data() -> ()  [unwired: 1 in, 5 out]
            n360 = property on="Scan rate voltage step priority" class="Bool (strict)"() -> ("Value"=w557:bool)  [unwired: 2 in, 2 out]
            n361 = case shown="True" w557 {
              frame False {
                n362 = property on="Scan rate measurement delay priority" class="Bool (strict)"("Value"=TRUE) -> ()  [unwired: 2 in, 2 out]
                n363 = property on="Step (V)" class="DigNum (strict)"("DisabledEnum"=T7."Disabled and Grayed Out" ("Disabled")) -> ()  [unwired: 2 in, 2 out]
                n364 = property on="Measurement delay (ms)" class="DigNum (strict)"("DisabledEnum"=T7."Enabled" ("Disabled")) -> ()  [unwired: 2 in, 2 out]
              }
              frame True {
                n365 = property on="Scan rate measurement delay priority" class="Bool (strict)"("Value"=FALSE) -> ()  [unwired: 2 in, 2 out]
                n366 = property on="Measurement delay (ms)" class="DigNum (strict)"("DisabledEnum"=T7."Disabled and Grayed Out" ("Disabled")) -> ()  [unwired: 2 in, 2 out]
                n367 = property on="Step (V)" class="DigNum (strict)"("DisabledEnum"=T7."Enabled" ("Disabled")) -> ()  [unwired: 2 in, 2 out]
              }
            }
          }
          event Value Change {
            n368 = event-data() -> ()  [unwired: 1 in, 5 out]
            n369 = property on="Scan rate measurement delay priority" class="Bool (strict)"() -> ("Value"=w568:bool)  [unwired: 2 in, 2 out]
            n370 = case shown="False" w568 {
              frame False {
                n371 = property on="Scan rate voltage step priority" class="Bool (strict)"("Value"=TRUE) -> ()  [unwired: 2 in, 2 out]
                n372 = property on="Measurement delay (ms)" class="DigNum (strict)"("DisabledEnum"=T7."Disabled and Grayed Out" ("Disabled")) -> ()  [unwired: 2 in, 2 out]
                n373 = property on="Step (V)" class="DigNum (strict)"("DisabledEnum"=T7."Enabled" ("Disabled")) -> ()  [unwired: 2 in, 2 out]
              }
              frame True {
                n374 = property on="Scan rate voltage step priority" class="Bool (strict)"("Value"=FALSE) -> ()  [unwired: 2 in, 2 out]
                n375 = property on="Measurement delay (ms)" class="DigNum (strict)"("DisabledEnum"=T7."Enabled" ("Disabled")) -> ()  [unwired: 2 in, 2 out]
                n376 = property on="Step (V)" class="DigNum (strict)"("DisabledEnum"=T7."Disabled and Grayed Out" ("Disabled")) -> ()  [unwired: 2 in, 2 out]
              }
            }
          }
          event Value Change {
            n377 = event-data() -> ()  [unwired: 1 in, 5 out]
            n378 = property on="Repeat light scans" class="Bool (strict)"() -> ("Value"=w579:bool)  [unwired: 2 in, 2 out]
            n379 = case shown="False" w579 {
              frame False {
                w580 = T7."Disabled and Grayed Out" ("Disabled")
                n380 = property on="No. of repeat scans" class="DigNum (strict)"("DisabledEnum"=w580) -> ()  [unwired: 2 in, 2 out]
                n381 = property on="Only repeat for best pixel" class="Ring (strict)"("DisabledEnum"=w580) -> ()  [unwired: 2 in, 2 out]
              }
              frame True {
                w581 = T7."Enabled" ("Disabled")
                n382 = property on="Only repeat for best pixel" class="Ring (strict)"("DisabledEnum"=w581) -> ()  [unwired: 2 in, 2 out]
                n383 = property on="No. of repeat scans" class="DigNum (strict)"("DisabledEnum"=w581) -> ()  [unwired: 2 in, 2 out]
              }
            }
          }
          event Value Change {
            n384 = event-data() -> ()  [unwired: 1 in, 5 out]
            n385 = property on="No. of scan rate steps" class="DigNum (strict)"() -> ("Value"=w585:dbl)  [unwired: 2 in, 2 out]
            n386 = property on="Scan rate measurement delay priority" class="Bool (strict)"() -> ("Value"=w596:bool)  [unwired: 2 in, 2 out]
            n387 = property on="J-V scan" class="Bool (strict)"() -> ("Value"=w591:bool)  [unwired: 2 in, 2 out]
            n388 = property on="Scan rate voltage step priority" class="Bool (strict)"() -> ("Value"=w597:bool)  [unwired: 2 in, 2 out]
            n389 = property on="Repeat light scans" class="Bool (strict)"() -> ("Value"=w582:bool)  [unwired: 2 in, 2 out]
            n390 = Greater?(x=w585, y=1.0) -> (0:w583:bool)
            n391 = property class="VI"() -> ("Panel"=w595:refnum<vi>)  [unwired: 2 in, 2 out]
            n392 = property on="Scan settings" class="Clust (strict)"() -> ("Controls[]"=w594:refnum<vi>[])  [unwired: 2 in, 2 out]
            n393 = local read "J-V cont. Lab.txt array"() -> (w593:string[])
            n394 = local read "J-V cond. cont. Lab.txt array"() -> (w592:string[])
            n395 = Build Array(w583, w597, w596, w582, w582) -> (w590:bool[])
            n396 = call "Disable-enable scan settgin controls.vi"("VI ref"=w595, "Scan settings control ref array"=w594, "Control Label.Text Array"=w593, "Cond. Control Label.Text Array"=w592, "Cond. Values array"=w590, "Enable?"=w591) -> ()  [unwired: 9 in, 1 out]
          }
          event Value Change {
            n397 = event-data() -> ()  [unwired: 1 in, 5 out]
            n398 = local read "J-t cont. Lab.txt array"() -> (w603:string[])
            n399 = property on="Scan settings" class="Clust (strict)"() -> ("Controls[]"=w604:refnum<vi>[])  [unwired: 2 in, 2 out]
            n400 = property class="VI"() -> ("Panel"=w605:refnum<vi>)  [unwired: 2 in, 2 out]
            n401 = property on="J-t scan" class="Bool (strict)"() -> ("Value"=w602:bool)  [unwired: 2 in, 2 out]
            n402 = call "Disable-enable scan settgin controls.vi"("VI ref"=w605, "Scan settings control ref array"=w604, "Control Label.Text Array"=w603, "Enable?"=w602) -> ()  [unwired: 11 in, 1 out]
          }
          event Value Change {
            n403 = event-data() -> ()  [unwired: 1 in, 5 out]
            n404 = property class="VI"() -> ("Panel"=w616:refnum<vi>)  [unwired: 2 in, 2 out]
            n405 = property on="Scan settings" class="Clust (strict)"() -> ("Controls[]"=w615:refnum<vi>[])  [unwired: 2 in, 2 out]
            n406 = local read "Max P cont. Lab.txt array"() -> (w613:string[])
            n407 = local read "Max P cond. cont. Lab.txt array"() -> (w612:string[])
            n408 = property on="Max P stab. Specific voltage" class="Bool (strict)"() -> ("Value"=w611:bool)  [unwired: 2 in, 2 out]
            n409 = property on="Max. power stabilisation" class="Bool (strict)"() -> ("Value"=w614:bool)  [unwired: 2 in, 2 out]
            n410 = Build Array(w611) -> (w610:bool[])
            n411 = call "Disable-enable scan settgin controls.vi"("VI ref"=w616, "Scan settings control ref array"=w615, "Control Label.Text Array"=w613, "Cond. Control Label.Text Array"=w612, "Cond. Values array"=w610, "Enable?"=w614) -> ()  [unwired: 9 in, 1 out]
          }
          event "Exit": Mouse Down {
            n412 = event-data() -> ()  [unwired: 1 in, 7 out]
            n413 = property on="Exit" class="Bool (strict)"() -> ("Value"=w617:bool)  [unwired: 2 in, 2 out]
          }
        }
      }
      frame "Measure" {
        (unwired) State_Enumerate_Ring."Idle" ("Enum")
        n414 = stacked-sequence {
          tunnel: w622 -> [_ _ _ _ w688 _ _]
          tunnel: [_ _ _ _ _ _ State_Enumerate_Ring."Notify" ("Enum")] -> w623
          tunnel: w622 -> [_ _ _ w653 w686 _ _]
          frame #0 {
            n415 = property on="Manual mode" class="Bool (strict)"() -> ("Value"=w626:bool)  [unwired: 2 in, 2 out]
            n416 = case shown="True" w626 {
              frame False {
                # "Move to diode"
                n417 = Two Button Dialog(message="Do you want to calibrate the lamp intensity?\n\n(If this is the first measurement click \"Yes\")", 1:"No" ("F button name (\"Cancel\")"), 2:"Yes" ("T button name (\"OK\")")) -> (T button?=w629:bool)
                "Calibrate?" <- w629
                n418 = case shown="True" w629 {
                  frame False {
                  }
                  frame True {
                    n419 = call "Move stage to diode position.vi"() -> ()  [unwired: 11 in, 1 out]
                  }
                }
              }
              frame True {
                w631 = u16 2 items=["PCB-Keithley", "PCB-EQE", "Manual-Keithley", "Manual-EQE"] ("Experiment type")
                n420 = local write "Calibrate?"(FALSE ("Calibrate?")) -> ()
                n421 = call "Set pins on switch board.vi"("Experiment type"=w631) -> ()  [unwired: 10 in, 1 out]
                n422 = local write "Experiment type"(w631) -> ()
              }
            }
          }
          frame #1 {
            n423 = property on="Manual mode" class="Bool (strict)"() -> ("Value"=w633:bool)  [unwired: 2 in, 2 out]
            n424 = case shown="False" w633 {
              frame False {
                # "Connect diode to Keithley"
                n425 = local read "Calibrate?"() -> (w634:bool)
                n426 = case shown="True" w634 {
                  frame False {
                  }
                  frame True {
                    n427 = call "Select pin on PCB.vi"("Pin"=128) -> ()  [unwired: 9 in, 1 out]
                  }
                }
              }
              frame True {
              }
            }
          }
          frame #2 {
            n428 = property on="Manual mode" class="Bool (strict)"() -> ("Value"=w636:bool)  [unwired: 2 in, 2 out]
            n429 = case shown="False" w636 {
              frame False {
                n430 = local read "Calibrate?"() -> (w637:bool)
                n431 = case shown="True" w637 {
                  frame False {
                  }
                  frame True {
                    # "Measure number of suns"
                    n432 = while {
                      stop <- w639 stop-if-true
                      n433 = call "Measure number of suns.vi"() -> ("Number of suns"=w650:dbl)  [unwired: 10 in, 1 out]
                      n434 = Number To Fractional String(number=w650) -> (F-format string=w638:string)  [unwired: 3 in]
                      "Number of suns" <- w638
                      n435 = Concatenate Strings("The lamp power is equivalent to ", w638, " suns.") -> (w648:string)
                      n436 = call <vilib>:"Three Button Dialog.vi"("Right Button Text (\"Cancel\")"="Abort", "Center Button Text (\"No\")"="Re-measure", "Left Button Text (\"Yes\")"="Proceed", "message"=w648) -> ("Which Button?"=w644:T8)  [unwired: 7 in]
                      n437 = Equal?(x=w644, y=0) -> (x = y?=w640:bool)
                      n438 = Equal?(x=w644, y=2) -> (x = y?=w641:bool)
                      "Abort" <- w641
                      n439 = Or(x=w640, y=w641) -> (x .or. y?=w639:bool)
                    }
                  }
                }
              }
              frame True {
              }
            }
          }
          frame #3 {
            # "If an intensity dependent measurement is to be performed, calibrate each filter wheel position i.e. measure number of suns for each filter"
            n440 = call "Build queue.vi"("Scan settings array"=w653, "Cell Settings Array"="Cell Settings Array 1") -> ("Measurement queue"=w662:T5)  [unwired: 9 in]
            "Measurement queue" <- w662
            n441 = for {
              tunnel: w662 -> [w685] mode=indexing
              tunnel: [w684] -> w661 mode=indexing
              n442 = Unbundle By Name(w685) -> ("Measurement type"=w684:string)
            }
            n443 = local read "Calibrate?"() -> (w656:bool)
            n444 = local read "Abort"() -> (w655:bool)
            n445 = Search 1D Array(1D array=w661, element="Intensity") -> (index of element=w659:i32)  [unwired: 1 in]
            n446 = Greater Or Equal To 0?(x=w659) -> (x >= 0?=w657:bool)
            n447 = Not(x=w655) -> (.not. x?=w654:bool)
            n448 = Compound Arithmetic op=AND(w657, w656, w654) -> (w658:bool)
            n449 = case shown="True" w658 {
              frame False {
              }
              frame True {
                n450 = call "Get filter wheel settings.vi"() -> ("All filter wheel settings"=w663:dbl[][], "Filter wheel numbers"=w664:dbl[], "Filter wheel settings file path"=w665:path)  [unwired: 7 in, 2 out]
                n451 = for {
                  tunnel: w664 -> [w681] mode=indexing
                  tunnel: w663 -> [w678]
                  tunnel: [w680] -> w675 mode=indexing
                  tunnel: [w678] -> w672
                  n452 = local read "Current Angle (degrees)"() -> (w677:dbl)
                  n453 = call "Get new anlge to rotate filter wheel by.vi"("Filter Wheel Positions"=w678, "Current anlge (degrees)"=w677, "Filter no."=w681) -> ("Clockwise?"=w682:bool, "Rotate by angle (degrees)"=w683:dbl, "New current anlge (degrees)"=w676:dbl)  [unwired: 6 in]
                  n454 = local write "Current Angle (degrees)"(w676) -> ()
                  n455 = call "Turn filter wheel by angle.vi"("Clockwise?"=w682, "Angle (degrees)"=w683) -> ("error out"=w679:errorcluster)  [unwired: 7 in, 2 out]
                  n456 = call "Measure number of suns.vi"("error in (no error)"=w679) -> ("Number of suns"=w680:dbl)  [unwired: 9 in, 1 out]
                }
                n457 = Replace Array Subset(array=w672, new element=w675, index (col)=2 ("disabled index (col)")) -> (w673:dbl[][])  [unwired: 1 in]
                n458 = local read "Current Angle (degrees)"() -> (w666:dbl)
                n459 = call-poly <vilib>:"Write To Spreadsheet File.vi"("2D data"=w673, "file path (dialog if empty)"=w665) -> ()  [unwired: 6 in, 1 out]
                n460 = call "Get new anlge to rotate filter wheel by.vi"("Filter Wheel Positions"=w672, "Current anlge (degrees)"=w666, "Filter no."=0.0) -> ("Clockwise?"=w670:bool, "Rotate by angle (degrees)"=w671:dbl)  [unwired: 6 in, 1 out]
                n461 = call "Turn filter wheel by angle.vi"("Clockwise?"=w670, "Angle (degrees)"=w671) -> ("Enable Channel out"=w668:u8, "Serial Port out"=w669:refnum<visa-resource-name>)  [unwired: 7 in, 1 out]
                n462 = call "Disable Motor.vi"("Enable Channel"=w668, "Serial Port"=w669) -> ()  [unwired: 9 in, 1 out]
              }
            }
          }
          frame #4 {
            n463 = local read "Abort"() -> (w687:bool)
            n464 = case shown="False" w687 {
              tunnel: w688 -> [w692 _]
              tunnel: w686 -> [w690 _]
              frame False {
                # "Run measurements"
                n465 = local read "Measurement queue"() -> (w689:T5)
                n466 = Get Date/Time In Seconds() -> (seconds since 1Jan1904=w693:timestamp)
                n467 = call "Timing Calculator_v2.vi"("Scan settings array"=w690, "Measurement queue"=w689) -> ("Experiment time (s)"=w691:dbl)  [unwired: 9 in]
                n468 = while {
                  tunnel: w693 -> [w700]
                  tunnel: w691 -> [w697]
                  stop <- w696 stop-if-true
                  n469 = call "Time left Calculator.vi"("Start time"=w700, "Experiment duration (s)"=w697) -> ("Finish time"=→"Finish time":timestamp, "Time Left"=→"Time left":dbl, "Time has Elapsed"=w695:bool)  [unwired: 6 in, 1 out]
                  n470 = local read "Scan stopped?"() -> (w694:bool)
                  n471 = Compound Arithmetic op=OR(w694, w695) -> (w696:bool)
                }
                n472 = while {
                  shift-right: [w702] -> _
                  shift-left: w689 -> [w708]
                  tunnel: w692 -> [w703]
                  stop <- w705 stop-if-true
                  n473 = Array Size(array=w708) -> (size(s)=w701:i32)
                  n474 = Equal?(x=0, y=w701) -> (x = y?=w706:bool)
                  n475 = Compound Arithmetic op=OR(w706, "Stop Scan 2") -> (w705:bool)
                  "Scan stopped?" <- w705
                  n476 = case shown="False" w705 {
                    tunnel: [w724 w1129] -> w702
                    tunnel: w708 -> [w723 w1129]
                    tunnel: w703 -> [w722 _]
                    frame False {
                      n477 = Delete From Array(array=w723, index=0) -> (deleted portion=w710:T9, array with subset deleted=w724:T5)  [unwired: 1 in]
                      n478 = Unbundle By Name(w710) -> ("Measurement type"=w714:string)
                      n479 = Unbundle By Name(w710) -> ("Scan settings in queue"=w720:u16)
                      n480 = call "Build meas status string.vi"("Cell details cluster in"=w710) -> ("Measurement status"=→"Measurement status:":string)  [unwired: 10 in]
                      n481 = Unbundle By Name(w710) -> ("Pixel to measure"=w715:u16)
                      n482 = Match Pattern(string=w714, regular expression=" - Scan rate ") -> (before substring=w712:string, after substring=w711:string)  [unwired: 1 in, 2 out]
                      n483 = Index Array(array=w722, index=w720) -> (element=w719:T3)
                      n484 = case shown="\"Intensity\"" w712 {
                        tunnel: w710 -> [w741 w801 w882 w939 w998 w1071]
                        tunnel: "User Name" -> [w740 w800 w881 w938 w997 w1074]
                        tunnel: "Experiment Title" -> [w739 w799 w880 w937 w996 w1073]
                        tunnel: w719 -> [w730 w793 w879 w936 w995 w1072]
                        tunnel: [w738 w806 w878 w935 w994 w1070] -> w718
                        tunnel: w715 -> [_ w791 w869 w926 w985 w1057]
                        tunnel: w711 -> [w733 w794 _ _ _ _]
                        frame "JV Scan", Default {
                          n485 = Unbundle By Name(w730) -> ("No. of scan rate steps"=w726:dbl)
                          n486 = Equal?(x=w726, y=1.0) -> (x = y?=w731:bool)
                          n487 = Decimal String To Number(string=w733) -> (number=w727:i32)  [unwired: 2 in, 1 out]
                          n488 = case shown="False" w731 {
                            tunnel: w730 -> [w747 w749]
                            tunnel: [w742 w748] -> w728
                            tunnel: w727 -> [w744 _]
                            tunnel: w726 -> [w743 _]
                            frame False {
                              n489 = Unbundle By Name(w747) -> ("Scan rate min (V/s)"=w746:dbl, "Scan rate max (V/s)"=w745:dbl)
                              n490 = call "Calculate scan rate.vi"("Scan rate number"=w744, "Number of steps"=w743, "Scan rate max (V/s)"=w745, "Scan rate min (V/s)"=w746) -> ("Scan rate"=w742:dbl)  [unwired: 7 in]
                            }
                            frame True {
                              n491 = Unbundle By Name(w749) -> ("Scan rate min (V/s)"=w748:dbl)
                            }
                          }
                          n492 = flat-sequence {
                            tunnel: [w752] -> w737
                            tunnel: [w755] -> w736
                            tunnel: [w754] -> w735
                            tunnel: [w753] -> w734
                            tunnel: w741 -> [w752]
                            tunnel: w740 -> [w755]
                            tunnel: w739 -> [w754]
                            tunnel: w730 -> [w753]
                            tunnel: [w751] -> w729
                            tunnel: w728 -> [w751]
                            tunnel: w737 -> [w777]
                            tunnel: w736 -> [w776]
                            tunnel: w735 -> [w775]
                            tunnel: w734 -> [w774]
                            tunnel: w729 -> [w770]
                            tunnel: [w772] -> w725
                            tunnel: [w781] -> w738
                            tunnel: w725 -> [w781]
                            frame #0 {
                              n493 = property on="Manual mode" class="Bool (strict)"() -> ("Value"=w750:bool)  [unwired: 2 in, 2 out]
                              n494 = case shown="True" w750 {
                                tunnel: w752 -> [w760 _]
                                frame False {
                                w758 = u16 0 items=["PCB-Keithley", "PCB-EQE", "Manual-Keithley", "Manual-EQE"] ("Experiment type")
                                n495 = local read "Experiment type"() -> (w757:u16)
                                n496 = Not Equal?(x=w757, y=w758) -> (x != y?=w756:bool)
                                n497 = case shown="True" w756 {
                                frame False {
                                }
                                frame True {
                                w763 = u16 0 items=["PCB-Keithley", "PCB-EQE", "Manual-Keithley", "Manual-EQE"] ("Experiment type")
                                n498 = local write "Experiment type"(w763) -> ()
                                n499 = call "Set pins on switch board.vi"("Experiment type"=w763) -> ()  [unwired: 10 in, 1 out]
                                }
                                }
                                n500 = call "Get pixel X-Y position.vi"("Cell Details Cluster"=w760) -> ("Pin"=w759:dbl, "Y position"=w762:string, "X position"=w761:string)  [unwired: 7 in]
                                n501 = call "Move X-Y to specific position.vi"("position 2"=w762, "position 1"=w761) -> ()  [unwired: 5 in, 5 out]
                                n502 = call "Select pin on PCB.vi"("Pin"=w759) -> ()  [unwired: 9 in, 1 out]
                                }
                                frame True {
                                w766 = u16 2 items=["PCB-Keithley", "PCB-EQE", "Manual-Keithley", "Manual-EQE"] ("Experiment type")
                                n503 = local read "Experiment type"() -> (w765:u16)
                                n504 = Not Equal?(x=w765, y=w766) -> (x != y?=w764:bool)
                                n505 = case shown="True" w764 {
                                frame False {
                                }
                                frame True {
                                w767 = u16 2 items=["PCB-Keithley", "PCB-EQE", "Manual-Keithley", "Manual-EQE"] ("Experiment type")
                                n506 = local write "Experiment type"(w767) -> ()
                                n507 = call "Set pins on switch board.vi"("Experiment type"=w767) -> ()  [unwired: 10 in, 1 out]
                                }
                                }
                                }
                              }
                            }
                            frame #1 {
                              n508 = local read "Number of suns"() -> (w769:string)
                              n509 = call "Measure JV curve.vi"("Skip pixel?"=FALSE, "Scan settings"=w774, "Cell details cluster"=w777, "Intensity (no. of suns)"=w769, "Scan rate (V/s)"=w770, "Experiment Title"=w775, "User Name"=w776) -> ("Log Table"=→"Log Table":string[][], "File path for master log"=→"File path for master log":path, "JV Curve"=w772:cluster{"Y":dbl[], "Y":dbl[]}[])  [unwired: 2 in]
                            }
                            frame #2 {
                              n510 = property on="JV Curve" class="XYGraph (strict)"("YScale.NameLbl.Text"="J (mA/cm^2)" ("Y Scale.Name Label.Text")) -> ()  [unwired: 2 in, 2 out]
                              n511 = for {
                                tunnel: string[] ["Scan 1", "Scan 2"] ("Measurement queue") -> [w782] mode=indexing
                                i -> [w783]
                                n512 = property on="JV Curve" class="XYGraph (strict)"("Active Plot"=w783, "Plot.Plot Name"=w782) -> ()  [unwired: 2 in, 2 out]
                              }
                              n513 = property on="JV Curve" class="XYGraph (strict)"("XScale.NameLbl.Text"="Applied Bias (V)" ("Y Scale.Name Label.Text")) -> ()  [unwired: 2 in, 2 out]
                            }
                          }
                        }
                        frame "Repeat JV Scan For Best" {
                          n514 = Unbundle By Name(w793) -> ("No. of scan rate steps"=w795:dbl)
                          n515 = Equal?(x=w795, y=1.0) -> (x = y?=w797:bool)
                          n516 = Decimal String To Number(string=w794) -> (number=w796:i32)  [unwired: 2 in, 1 out]
                          n517 = case shown="False" w797 {
                            tunnel: w793 -> [w817 w820]
                            tunnel: [w812 w819] -> w788
                            tunnel: w796 -> [w814 _]
                            tunnel: w795 -> [w813 _]
                            tunnel: [w811 w818] -> w792
                            tunnel: w791 -> [w811 w818]
                            frame False {
                              n518 = Unbundle By Name(w817) -> ("Scan rate min (V/s)"=w816:dbl, "Scan rate max (V/s)"=w815:dbl)
                              n519 = call "Calculate scan rate.vi"("Scan rate number"=w814, "Number of steps"=w813, "Scan rate max (V/s)"=w815, "Scan rate min (V/s)"=w816) -> ("Scan rate"=w812:dbl)  [unwired: 7 in]
                            }
                            frame True {
                              n520 = Unbundle By Name(w820) -> ("Scan rate min (V/s)"=w819:dbl)
                            }
                          }
                          n521 = flat-sequence {
                            tunnel: w793 -> [w828]
                            tunnel: w799 -> [w829]
                            tunnel: w800 -> [w830]
                            tunnel: w801 -> [w826]
                            tunnel: [w825] -> w805
                            tunnel: [w830] -> w804
                            tunnel: [w829] -> w803
                            tunnel: [w828] -> w802
                            tunnel: w792 -> [w824]
                            tunnel: [w823] -> w789
                            tunnel: w788 -> [w823]
                            tunnel: [w822] -> w785
                            tunnel: [w821] -> w784
                            tunnel: [w834] -> w810
                            tunnel: [w837] -> w809
                            tunnel: [w836] -> w808
                            tunnel: [w835] -> w807
                            tunnel: w805 -> [w834]
                            tunnel: w804 -> [w837]
                            tunnel: w803 -> [w836]
                            tunnel: w802 -> [w835]
                            tunnel: [w833] -> w790
                            tunnel: w789 -> [w833]
                            tunnel: [w832] -> w786
                            tunnel: w785 -> [w832]
                            tunnel: w784 -> [w831]
                            tunnel: w810 -> [w858]
                            tunnel: w809 -> [w857]
                            tunnel: w808 -> [w856]
                            tunnel: w807 -> [w855]
                            tunnel: w790 -> [w851]
                            tunnel: [w854] -> w787
                            tunnel: w786 -> [w850]
                            tunnel: [w862] -> w806
                            tunnel: w787 -> [w862]
                            frame #0 {
                              n522 = local read "File path for master log"() -> (w827:path)
                              n523 = property on="Manual mode" class="Bool (strict)"() -> ("Value"=w821:bool)  [unwired: 2 in, 2 out]
                              n524 = call "Find best pixel from log file.vi"("Manual mode?"=w821, "Cell details cluster in"=w826, "Nth best pixel"=w824, "File path of JV log"=w827) -> ("Skip pixel?"=w822:bool, "Best pixel cell details cluster"=w825:T9)  [unwired: 6 in]
                            }
                            frame #1 {
                              n525 = case shown="True" w831 {
                                tunnel: w834 -> [w841 _]
                                frame False {
                                w839 = u16 0 items=["PCB-Keithley", "PCB-EQE", "Manual-Keithley", "Manual-EQE"] ("Experiment type")
                                n526 = local read "Experiment type"() -> (w838:u16)
                                n527 = call "Get pixel X-Y position.vi"("Cell Details Cluster"=w841) -> ("Pin"=w844:dbl, "Y position"=w843:string, "X position"=w842:string)  [unwired: 7 in]
                                n528 = call "Move X-Y to specific position.vi"("position 2"=w843, "position 1"=w842) -> ()  [unwired: 5 in, 5 out]
                                n529 = call "Select pin on PCB.vi"("Pin"=w844) -> ()  [unwired: 9 in, 1 out]
                                n530 = Not Equal?(x=w838, y=w839) -> (x != y?=w840:bool)
                                n531 = case shown="True" w840 {
                                frame False {
                                }
                                frame True {
                                w845 = u16 0 items=["PCB-Keithley", "PCB-EQE", "Manual-Keithley", "Manual-EQE"] ("Experiment type")
                                n532 = call "Set pins on switch board.vi"("Experiment type"=w845) -> ()  [unwired: 10 in, 1 out]
                                n533 = local write "Experiment type"(w845) -> ()
                                }
                                }
                                }
                                frame True {
                                w847 = u16 2 items=["PCB-Keithley", "PCB-EQE", "Manual-Keithley", "Manual-EQE"] ("Experiment type")
                                n534 = local read "Experiment type"() -> (w848:u16)
                                n535 = Not Equal?(x=w848, y=w847) -> (x != y?=w846:bool)
                                n536 = case shown="True" w846 {
                                frame False {
                                }
                                frame True {
                                w849 = u16 2 items=["PCB-Keithley", "PCB-EQE", "Manual-Keithley", "Manual-EQE"] ("Experiment type")
                                n537 = call "Set pins on switch board.vi"("Experiment type"=w849) -> ()  [unwired: 10 in, 1 out]
                                n538 = local write "Experiment type"(w849) -> ()
                                }
                                }
                                }
                              }
                            }
                            frame #2 {
                              n539 = local read "Number of suns"() -> (w852:string)
                              n540 = call "Measure JV curve.vi"("Skip pixel?"=w850, "Scan settings"=w855, "Cell details cluster"=w858, "Intensity (no. of suns)"=w852, "Scan rate (V/s)"=w851, "Experiment Title"=w856, "User Name"=w857) -> ("Log Table"=w853:string[][], "JV Curve"=w854:cluster{"Y":dbl[], "Y":dbl[]}[])  [unwired: 2 in, 1 out]
                              n541 = local write "Log Table"(w853) -> ()
                            }
                            frame #3 {
                              n542 = for {
                                tunnel: string[] ["Scan 1", "Scan 2"] ("Measurement queue") -> [w863] mode=indexing
                                i -> [w864]
                                n543 = property on="JV Curve" class="XYGraph (strict)"("Active Plot"=w864, "Plot.Plot Name"=w863) -> ()  [unwired: 2 in, 2 out]
                              }
                              n544 = property on="JV Curve" class="XYGraph (strict)"("XScale.NameLbl.Text"="Applied Bias (V)" ("Y Scale.Name Label.Text")) -> ()  [unwired: 2 in, 2 out]
                              n545 = property on="JV Curve" class="XYGraph (strict)"("YScale.NameLbl.Text"="J (mA/cm^2)" ("Y Scale.Name Label.Text")) -> ()  [unwired: 2 in, 2 out]
                            }
                          }
                        }
                        frame "Jt Scan" {
                          n546 = flat-sequence {
                            tunnel: w879 -> [w889]
                            tunnel: w880 -> [w890]
                            tunnel: w881 -> [w891]
                            tunnel: w882 -> [w886]
                            tunnel: [w885] -> w873
                            tunnel: [w891] -> w872
                            tunnel: [w890] -> w871
                            tunnel: [w889] -> w870
                            tunnel: w869 -> [w887]
                            tunnel: [w884] -> w866
                            tunnel: [w883] -> w865
                            tunnel: [w894] -> w877
                            tunnel: [w897] -> w876
                            tunnel: [w896] -> w875
                            tunnel: [w895] -> w874
                            tunnel: w873 -> [w894]
                            tunnel: w872 -> [w897]
                            tunnel: w871 -> [w896]
                            tunnel: w870 -> [w895]
                            tunnel: [w893] -> w867
                            tunnel: w866 -> [w893]
                            tunnel: w865 -> [w892]
                            tunnel: w877 -> [w915]
                            tunnel: w876 -> [w914]
                            tunnel: w875 -> [w913]
                            tunnel: w874 -> [w912]
                            tunnel: [w911] -> w868
                            tunnel: w867 -> [w910]
                            tunnel: [w919] -> w878
                            tunnel: w868 -> [w919]
                            frame #0 {
                              n547 = local read "File path for master log"() -> (w888:path)
                              n548 = property on="Manual mode" class="Bool (strict)"() -> ("Value"=w883:bool)  [unwired: 2 in, 2 out]
                              n549 = call "Find best pixel from log file.vi"("Manual mode?"=w883, "Cell details cluster in"=w886, "Nth best pixel"=w887, "File path of JV log"=w888) -> ("Skip pixel?"=w884:bool, "Best pixel cell details cluster"=w885:T9)  [unwired: 6 in]
                            }
                            frame #1 {
                              n550 = case shown="True" w892 {
                                tunnel: w894 -> [w901 _]
                                frame False {
                                w900 = u16 0 items=["PCB-Keithley", "PCB-EQE", "Manual-Keithley", "Manual-EQE"] ("Experiment type")
                                n551 = local read "Experiment type"() -> (w899:u16)
                                n552 = Not Equal?(x=w899, y=w900) -> (x != y?=w898:bool)
                                n553 = call "Get pixel X-Y position.vi"("Cell Details Cluster"=w901) -> ("Pin"=w904:dbl, "Y position"=w903:string, "X position"=w902:string)  [unwired: 7 in]
                                n554 = case shown="True" w898 {
                                frame False {
                                }
                                frame True {
                                w905 = u16 0 items=["PCB-Keithley", "PCB-EQE", "Manual-Keithley", "Manual-EQE"] ("Experiment type")
                                n555 = call "Set pins on switch board.vi"("Experiment type"=w905) -> ()  [unwired: 10 in, 1 out]
                                n556 = local write "Experiment type"(w905) -> ()
                                }
                                }
                                n557 = call "Move X-Y to specific position.vi"("position 2"=w903, "position 1"=w902) -> ()  [unwired: 5 in, 5 out]
                                n558 = call "Select pin on PCB.vi"("Pin"=w904) -> ()  [unwired: 9 in, 1 out]
                                }
                                frame True {
                                w908 = u16 2 items=["PCB-Keithley", "PCB-EQE", "Manual-Keithley", "Manual-EQE"] ("Experiment type")
                                n559 = local read "Experiment type"() -> (w907:u16)
                                n560 = Not Equal?(x=w907, y=w908) -> (x != y?=w906:bool)
                                n561 = case shown="True" w906 {
                                frame False {
                                }
                                frame True {
                                w909 = u16 2 items=["PCB-Keithley", "PCB-EQE", "Manual-Keithley", "Manual-EQE"] ("Experiment type")
                                n562 = call "Set pins on switch board.vi"("Experiment type"=w909) -> ()  [unwired: 10 in, 1 out]
                                n563 = local write "Experiment type"(w909) -> ()
                                }
                                }
                                }
                              }
                            }
                            frame #2 {
                              n564 = call "Measure Jt curve.vi"("Skip pixel?"=w910, "Scan settings"=w912, "Cell details cluster"=w915, "Experiment Title"=w913, "User Name"=w914) -> ("Jt Curve"=w911:cluster{"Y":dbl[], "Y":dbl[]}[])  [unwired: 6 in]
                            }
                            frame #3 {
                              n565 = for {
                                tunnel: string[] ["Scan 1", "Scan 2"] ("Measurement queue") -> [w920] mode=indexing
                                i -> [w921]
                                n566 = property on="JV Curve" class="XYGraph (strict)"("Active Plot"=w921, "Plot.Plot Name"=w920) -> ()  [unwired: 2 in, 2 out]
                              }
                              n567 = property on="JV Curve" class="XYGraph (strict)"("YScale.NameLbl.Text"="J (mA/cm^2)" ("Y Scale.Name Label.Text")) -> ()  [unwired: 2 in, 2 out]
                              n568 = property on="JV Curve" class="XYGraph (strict)"("XScale.NameLbl.Text"="Time (s)" ("Y Scale.Name Label.Text")) -> ()  [unwired: 2 in, 2 out]
                            }
                          }
                        }
                        frame "Max P Stabilization" {
                          n569 = flat-sequence {
                            tunnel: w936 -> [w946]
                            tunnel: w937 -> [w947]
                            tunnel: w938 -> [w948]
                            tunnel: w939 -> [w945]
                            tunnel: [w944] -> w930
                            tunnel: [w948] -> w929
                            tunnel: [w947] -> w928
                            tunnel: [w946] -> w927
                            tunnel: w926 -> [w942]
                            tunnel: [w941] -> w923
                            tunnel: [w940] -> w922
                            tunnel: [w951] -> w934
                            tunnel: [w954] -> w933
                            tunnel: [w953] -> w932
                            tunnel: [w952] -> w931
                            tunnel: w930 -> [w951]
                            tunnel: w929 -> [w954]
                            tunnel: w928 -> [w953]
                            tunnel: w927 -> [w952]
                            tunnel: [w950] -> w924
                            tunnel: w923 -> [w950]
                            tunnel: w922 -> [w949]
                            tunnel: w934 -> [w974]
                            tunnel: w933 -> [w973]
                            tunnel: w932 -> [w972]
                            tunnel: w931 -> [w971]
                            tunnel: [w970] -> w925
                            tunnel: w924 -> [w967]
                            tunnel: [w978] -> w935
                            tunnel: w925 -> [w978]
                            frame #0 {
                              n570 = local read "File path for master log"() -> (w943:path)
                              n571 = property on="Manual mode" class="Bool (strict)"() -> ("Value"=w940:bool)  [unwired: 2 in, 2 out]
                              n572 = call "Find best pixel from log file.vi"("Manual mode?"=w940, "Cell details cluster in"=w945, "Nth best pixel"=w942, "File path of JV log"=w943) -> ("Skip pixel?"=w941:bool, "Best pixel cell details cluster"=w944:T9)  [unwired: 6 in]
                            }
                            frame #1 {
                              n573 = case shown="True" w949 {
                                tunnel: w951 -> [w958 _]
                                frame False {
                                w957 = u16 0 items=["PCB-Keithley", "PCB-EQE", "Manual-Keithley", "Manual-EQE"] ("Experiment type")
                                n574 = local read "Experiment type"() -> (w956:u16)
                                n575 = call "Get pixel X-Y position.vi"("Cell Details Cluster"=w958) -> ("Pin"=w961:dbl, "Y position"=w960:string, "X position"=w959:string)  [unwired: 7 in]
                                n576 = Not Equal?(x=w956, y=w957) -> (x != y?=w955:bool)
                                n577 = call "Move X-Y to specific position.vi"("position 2"=w960, "position 1"=w959) -> ()  [unwired: 5 in, 5 out]
                                n578 = call "Select pin on PCB.vi"("Pin"=w961) -> ()  [unwired: 9 in, 1 out]
                                n579 = case shown="True" w955 {
                                frame False {
                                }
                                frame True {
                                w962 = u16 0 items=["PCB-Keithley", "PCB-EQE", "Manual-Keithley", "Manual-EQE"] ("Experiment type")
                                n580 = call "Set pins on switch board.vi"("Experiment type"=w962) -> ()  [unwired: 10 in, 1 out]
                                n581 = local write "Experiment type"(w962) -> ()
                                }
                                }
                                }
                                frame True {
                                w964 = u16 2 items=["PCB-Keithley", "PCB-EQE", "Manual-Keithley", "Manual-EQE"] ("Experiment type")
                                n582 = local read "Experiment type"() -> (w965:u16)
                                n583 = Not Equal?(x=w965, y=w964) -> (x != y?=w963:bool)
                                n584 = case shown="True" w963 {
                                frame False {
                                }
                                frame True {
                                w966 = u16 2 items=["PCB-Keithley", "PCB-EQE", "Manual-Keithley", "Manual-EQE"] ("Experiment type")
                                n585 = call "Set pins on switch board.vi"("Experiment type"=w966) -> ()  [unwired: 10 in, 1 out]
                                n586 = local write "Experiment type"(w966) -> ()
                                }
                                }
                                }
                              }
                            }
                            frame #2 {
                              n587 = local read "Number of suns"() -> (w968:string)
                              n588 = local read "File path for master log"() -> (w969:path)
                              n589 = call "Measure MaxPStabilisation.vi"("Skip pixel?"=w967, "Scan settings"=w971, "Cell details cluster"=w974, "Intensity (no. of suns)"=w968, "File path of JV log"=w969, "Experiment Title"=w972, "User Name"=w973) -> ("Jt Curve"=w970:cluster{"Y":dbl[], "Y":dbl[]}[])  [unwired: 4 in]
                            }
                            frame #3 {
                              n590 = property on="JV Curve" class="XYGraph (strict)"("XScale.NameLbl.Text"="Time (s)" ("Y Scale.Name Label.Text")) -> ()  [unwired: 2 in, 2 out]
                              n591 = for {
                                tunnel: string[] ["|PCE (%)|", "|J (mA/cm^2)|"] ("Measurement queue") -> [w979] mode=indexing
                                i -> [w980]
                                n592 = property on="JV Curve" class="XYGraph (strict)"("Active Plot"=w980, "Plot.Plot Name"=w979) -> ()  [unwired: 2 in, 2 out]
                              }
                              n593 = property on="JV Curve" class="XYGraph (strict)"("YScale.NameLbl.Text"="|PCE (%)| or |J (mA/cm^2)|" ("Y Scale.Name Label.Text")) -> ()  [unwired: 2 in, 2 out]
                            }
                          }
                        }
                        frame "Intensity" {
                          n594 = flat-sequence {
                            tunnel: w995 -> [w1005]
                            tunnel: w996 -> [w1006]
                            tunnel: w997 -> [w1007]
                            tunnel: w998 -> [w1004]
                            tunnel: [w1003] -> w989
                            tunnel: [w1007] -> w988
                            tunnel: [w1006] -> w987
                            tunnel: [w1005] -> w986
                            tunnel: w985 -> [w1001]
                            tunnel: [w1000] -> w983
                            tunnel: [w999] -> w982
                            tunnel: [w1010] -> w993
                            tunnel: [w1013] -> w992
                            tunnel: [w1012] -> w991
                            tunnel: [w1011] -> w990
                            tunnel: w989 -> [w1010]
                            tunnel: w988 -> [w1013]
                            tunnel: w987 -> [w1012]
                            tunnel: w986 -> [w1011]
                            tunnel: w983 -> [w1009]
                            tunnel: w982 -> [w1008]
                            tunnel: [w1008] -> w981
                            tunnel: w993 -> [w1033]
                            tunnel: w992 -> [w1032]
                            tunnel: w991 -> [w1031]
                            tunnel: w990 -> [w1030]
                            tunnel: [w1029] -> w984
                            tunnel: w981 -> [w1026]
                            tunnel: [w1049] -> w994
                            tunnel: w984 -> [w1049]
                            frame #0 {
                              n595 = local read "File path for master log"() -> (w1002:path)
                              n596 = property on="Manual mode" class="Bool (strict)"() -> ("Value"=w1000:bool)  [unwired: 2 in, 2 out]
                              n597 = call "Find best pixel from log file.vi"("Manual mode?"=w1000, "Cell details cluster in"=w1004, "Nth best pixel"=w1001, "File path of JV log"=w1002) -> ("Skip pixel?"=w999:bool, "Best pixel cell details cluster"=w1003:T9)  [unwired: 6 in]
                            }
                            frame #1 {
                              n598 = case shown="True" w1009 {
                                tunnel: w1010 -> [w1017 _]
                                frame False {
                                w1016 = u16 0 items=["PCB-Keithley", "PCB-EQE", "Manual-Keithley", "Manual-EQE"] ("Experiment type")
                                n599 = local read "Experiment type"() -> (w1015:u16)
                                n600 = Not Equal?(x=w1015, y=w1016) -> (x != y?=w1014:bool)
                                n601 = call "Get pixel X-Y position.vi"("Cell Details Cluster"=w1017) -> ("Pin"=w1020:dbl, "Y position"=w1019:string, "X position"=w1018:string)  [unwired: 7 in]
                                n602 = case shown="True" w1014 {
                                frame False {
                                }
                                frame True {
                                w1021 = u16 0 items=["PCB-Keithley", "PCB-EQE", "Manual-Keithley", "Manual-EQE"] ("Experiment type")
                                n603 = call "Set pins on switch board.vi"("Experiment type"=w1021) -> ()  [unwired: 10 in, 1 out]
                                n604 = local write "Experiment type"(w1021) -> ()
                                }
                                }
                                n605 = call "Move X-Y to specific position.vi"("position 2"=w1019, "position 1"=w1018) -> ()  [unwired: 5 in, 5 out]
                                n606 = call "Select pin on PCB.vi"("Pin"=w1020) -> ()  [unwired: 9 in, 1 out]
                                }
                                frame True {
                                w1023 = u16 2 items=["PCB-Keithley", "PCB-EQE", "Manual-Keithley", "Manual-EQE"] ("Experiment type")
                                n607 = local read "Experiment type"() -> (w1024:u16)
                                n608 = Not Equal?(x=w1024, y=w1023) -> (x != y?=w1022:bool)
                                n609 = case shown="True" w1022 {
                                frame False {
                                }
                                frame True {
                                w1025 = u16 2 items=["PCB-Keithley", "PCB-EQE", "Manual-Keithley", "Manual-EQE"] ("Experiment type")
                                n610 = call "Set pins on switch board.vi"("Experiment type"=w1025) -> ()  [unwired: 10 in, 1 out]
                                n611 = local write "Experiment type"(w1025) -> ()
                                }
                                }
                                }
                              }
                            }
                            frame #2 {
                              n612 = call "Get filter wheel settings.vi"("Skip pixel"=w1026) -> ("Filter intensities"=w1027:dbl[], "Filter wheel numbers"=w1028:dbl[])  [unwired: 6 in, 3 out]
                              n613 = for {
                                tunnel: w1033 -> [w1045]
                                tunnel: w1032 -> [w1044]
                                tunnel: w1031 -> [w1043]
                                tunnel: w1030 -> [w1042]
                                tunnel: [w1041] -> w1029
                                tunnel: w1028 -> [w1038] mode=indexing
                                tunnel: w1027 -> [w1037] mode=indexing
                                tunnel: w1026 -> [w1034]
                                n614 = local read "Current Angle (degrees)"() -> (w1039:dbl)
                                n615 = call "Move to filter position.vi"("Current anlge (degrees)"=w1039, "Filter no."=w1038) -> ("error out"=w1035:errorcluster, "New current anlge (degrees)"=w1036:dbl)  [unwired: 8 in]
                                n616 = local write "Current Angle (degrees)"(w1036) -> ()
                                n617 = call "Measure Intensity Dep.vi"("User Name"=w1044, "Cell details cluster"=w1045, "Experiment Title"=w1043, "No. of Suns"=w1037, "error in (no error)"=w1035, "Scan settings"=w1042, "Skip pixel?"=w1034) -> ("JV Curve"=w1041:cluster{"Y":dbl[], "Y":dbl[]}[], "Log Table"=w1040:string[][])  [unwired: 7 in]
                                n618 = local write "Log Table"(w1040) -> ()
                              }
                            }
                            frame #3 {
                              n619 = for {
                                tunnel: string[] ["Scan 1", "Scan 2"] ("Measurement queue") -> [w1050] mode=indexing
                                i -> [w1051]
                                n620 = property on="JV Curve" class="XYGraph (strict)"("Active Plot"=w1051, "Plot.Plot Name"=w1050) -> ()  [unwired: 2 in, 2 out]
                              }
                              n621 = property on="JV Curve" class="XYGraph (strict)"("YScale.NameLbl.Text"="J (mA/cm^2)" ("Y Scale.Name Label.Text")) -> ()  [unwired: 2 in, 2 out]
                              n622 = property on="JV Curve" class="XYGraph (strict)"("XScale.NameLbl.Text"="Applied Bias (V)" ("Y Scale.Name Label.Text")) -> ()  [unwired: 2 in, 2 out]
                            }
                          }
                        }
                        frame "EQE" {
                          n623 = flat-sequence {
                            tunnel: w1071 -> [w1080]
                            tunnel: w1072 -> [w1081]
                            tunnel: w1073 -> [w1082]
                            tunnel: w1074 -> [w1083]
                            tunnel: [w1083] -> w1061
                            tunnel: [w1082] -> w1060
                            tunnel: [w1081] -> w1059
                            tunnel: [w1079] -> w1058
                            tunnel: w1057 -> [w1077]
                            tunnel: [w1076] -> w1055
                            tunnel: [w1075] -> w1054
                            tunnel: [w1089] -> w1065
                            tunnel: [w1088] -> w1064
                            tunnel: [w1087] -> w1063
                            tunnel: [w1086] -> w1062
                            tunnel: w1061 -> [w1089]
                            tunnel: w1060 -> [w1088]
                            tunnel: w1059 -> [w1087]
                            tunnel: w1058 -> [w1086]
                            tunnel: w1055 -> [w1085]
                            tunnel: w1054 -> [w1084]
                            tunnel: [w1084] -> w1053
                            tunnel: [w1109] -> w1069
                            tunnel: [w1108] -> w1068
                            tunnel: [w1107] -> w1067
                            tunnel: [w1106] -> w1066
                            tunnel: w1065 -> [w1109]
                            tunnel: w1064 -> [w1108]
                            tunnel: w1063 -> [w1107]
                            tunnel: w1062 -> [w1106]
                            tunnel: w1053 -> [w1102]
                            tunnel: [w1102] -> w1052
                            tunnel: w1069 -> [w1123]
                            tunnel: w1068 -> [w1122]
                            tunnel: w1067 -> [w1114]
                            tunnel: w1066 -> [w1112]
                            tunnel: [w1111] -> w1056
                            tunnel: w1052 -> [w1110]
                            tunnel: [w1128] -> w1070
                            tunnel: w1056 -> [w1128]
                            frame #0 {
                              n624 = local read "File path for master log"() -> (w1078:path)
                              n625 = property on="Manual mode" class="Bool (strict)"() -> ("Value"=w1076:bool)  [unwired: 2 in, 2 out]
                              n626 = call "Find best pixel from log file.vi"("Manual mode?"=w1076, "Cell details cluster in"=w1080, "Nth best pixel"=w1077, "File path of JV log"=w1078) -> ("Skip pixel?"=w1075:bool, "Best pixel cell details cluster"=w1079:T9)  [unwired: 6 in]
                            }
                            frame #1 {
                              n627 = case shown="True" w1085 {
                                tunnel: w1086 -> [w1093 _]
                                frame False {
                                w1091 = u16 1 items=["PCB-Keithley", "PCB-EQE", "Manual-Keithley", "Manual-EQE"] ("Experiment type")
                                n628 = local read "Experiment type"() -> (w1092:u16)
                                n629 = call "Get pixel X-Y position.vi"("Cell Details Cluster"=w1093) -> ("Pin"=w1096:dbl, "Y position"=w1095:string, "X position"=w1094:string)  [unwired: 7 in]
                                n630 = Not Equal?(x=w1092, y=w1091) -> (x != y?=w1090:bool)
                                n631 = call "Move X-Y to specific position.vi"("position 2"=w1095, "position 1"=w1094) -> ()  [unwired: 5 in, 5 out]
                                n632 = call "Select pin on PCB.vi"("Pin"=w1096) -> ()  [unwired: 9 in, 1 out]
                                n633 = case shown="True" w1090 {
                                frame False {
                                }
                                frame True {
                                w1097 = u16 1 items=["PCB-Keithley", "PCB-EQE", "Manual-Keithley", "Manual-EQE"] ("Experiment type")
                                n634 = call "Set pins on switch board.vi"("Experiment type"=w1097) -> ()  [unwired: 10 in, 1 out]
                                n635 = local write "Experiment type"(w1097) -> ()
                                }
                                }
                                }
                                frame True {
                                w1100 = u16 3 items=["PCB-Keithley", "PCB-EQE", "Manual-Keithley", "Manual-EQE"] ("Experiment type")
                                n636 = local read "Experiment type"() -> (w1099:u16)
                                n637 = Not Equal?(x=w1099, y=w1100) -> (x != y?=w1098:bool)
                                n638 = case shown="True" w1098 {
                                frame False {
                                }
                                frame True {
                                w1101 = u16 3 items=["PCB-Keithley", "PCB-EQE", "Manual-Keithley", "Manual-EQE"] ("Experiment type")
                                n639 = call "Set pins on switch board.vi"("Experiment type"=w1101) -> ()  [unwired: 10 in, 1 out]
                                n640 = local write "Experiment type"(w1101) -> ()
                                }
                                }
                                }
                              }
                            }
                            frame #2 {
                              n641 = local read "Current Angle (degrees)"() -> (w1105:dbl)
                              n642 = call "Move to filter position.vi"("Skip cell?"=w1102, "Current anlge (degrees)"=w1105, "Filter no."=10.0) -> ("New current anlge (degrees)"=w1104:dbl)  [unwired: 7 in, 1 out]
                              n643 = local write "Current Angle (degrees)"(w1104) -> ()
                            }
                            frame #3 {
                              n644 = call "Create EQE Data Folder and File Path.vi"("Skip cell?"=w1110, "Cell details cluster"=w1112, "Experiment Indicator"=w1122, "username"=w1123) -> ("EQE data file path string"=w1121:string, "EQE Data Output Folder"=w1115:path)  [unwired: 5 in, 1 out]
                              n645 = call "Measure EQE.vi"("Skip cell?"=w1110, "Scan settings"=w1114, "Save data file path"=w1121) -> ("Max WL (nm)"=w1118:string, "Min WL (nm)"=w1119:string, "EQE data file path"=w1120:path)  [unwired: 6 in]
                              n646 = call "CalculateEQEandJsc.vi"("Skip cell?"=w1110, "Cell details cluster"=w1112, "Max WL"=w1118, "Min WL"=w1119, "Pixel meas file path"=w1120) -> ("Mismatch factor"=w1116:dbl, "Jsc at 1 sun (mA/cm^2)"=w1117:dbl, "EQE file path"=w1113:path)  [unwired: 4 in]
                              n647 = call "Add Data to EQE Log File.vi"("Skip cell?"=w1110, "Scan settings"=w1114, "Cell details cluster"=w1112, "EQE Data Output Folder"=w1115, "Mismatch Factor"=w1116, "Jsc @ 1 sun (mA/cm^2)"=w1117, "File path for EQE data"=w1113) -> ("EQE Curve"=w1111:cluster{"all rows":dbl[], "all rows":dbl[]}[])  [unwired: 1 in, 3 out]
                            }
                            frame #4 {
                              n648 = property on="JV Curve" class="XYGraph (strict)"("YScale.NameLbl.Text"="EQE (%)" ("Y Scale.Name Label.Text")) -> ()  [unwired: 2 in, 2 out]
                              n649 = property on="JV Curve" class="XYGraph (strict)"("XScale.NameLbl.Text"="Wavelength (nm)" ("Y Scale.Name Label.Text")) -> ()  [unwired: 2 in, 2 out]
                              n650 = property on="JV Curve" class="XYGraph (strict)"("Active Plot"=u32 0, "Plot.Plot Name"="EQE") -> ()  [unwired: 2 in, 2 out]
                            }
                          }
                        }
                      }
                      "JV Curve" <- w718
                    }
                    frame True {
                    }
                  }
                  n651 = local write "Measurement queue"(w702) -> ()
                }
              }
              frame True {
              }
            }
          }
          frame #5 {
            n652 = property on="Manual mode" class="Bool (strict)"() -> ("Value"=w1130:bool)  [unwired: 2 in, 2 out]
            n653 = case shown="False" w1130 {
              frame False {
                # "Move to load position"
                n654 = Concatenate Strings("X", "10000") -> (w1134:string)
                n655 = Concatenate Strings("Y", "20000") -> (w1133:string)
                n656 = call "Move X-Y to specific position.vi"("position 2"=w1133, "position 1"=w1134) -> ()  [unwired: 5 in, 5 out]
              }
              frame True {
              }
            }
          }
          frame #6 {
          }
        }
        n657 = property on="Exit program" class="Bool (strict)"("DisabledEnum"=T7."Disabled and Grayed Out" ("Disabled")) -> ()  [unwired: 2 in, 2 out]
      }
      frame "Notify" {
        n658 = property on="Manual mode" class="Bool (strict)"() -> ("Value"=w1138:bool)  [unwired: 2 in, 2 out]
        n659 = case shown="False" w1138 {
          tunnel: [w1143 State_Enumerate_Ring."Idle" ("Enum")] -> w1140
          frame False {
            n660 = flat-sequence {
              tunnel: [State_Enumerate_Ring."Idle" ("Enum")] -> w1143
              frame #0 {
                w1144 = "Analysing data..." ("Status:")
                n661 = local write "Measurement status:"(w1144) -> ()
                n662 = local write "Status:"(w1144) -> ()
              }
              frame #1 {
                n663 = local read "Experiment Title"() -> (w1145:string)
                n664 = local read "File path for master log"() -> (w1146:path)
                n665 = call "JV Data analysis from master log file.vi"("Experiment Indicator"=w1145, "Master log filepath"=w1146) -> ()  [unwired: 10 in]
              }
              frame #2 {
                n666 = local write "Measurement status:"("") -> ()
                n667 = local write "Status:"("Ready!" ("Status:")) -> ()
              }
              frame #3 {
                n668 = One Button Dialog(message="Experiment complete!") -> ()  [unwired: 1 in, 1 out]
              }
              frame #4 {
                n669 = local read "Init/idle Lab.txt array"() -> (w1153:string[])
                n670 = property class="VI"() -> (error out=w1152:errorcluster, "Panel"=w1151:refnum<vi>)  [unwired: 2 in, 1 out]
                n671 = call "Disable and grey out controls.vi"("Control Label.Text Array"=w1153, "error in (no error)"=w1152, "VI ref"=w1151) -> ()  [unwired: 9 in]
              }
            }
          }
          frame True {
            n672 = local read "Init/idle Lab.txt array"() -> (w1154:string[])
            n673 = property class="VI"() -> (error out=w1156:errorcluster, "Panel"=w1157:refnum<vi>)  [unwired: 2 in, 1 out]
            n674 = call "Disable and grey out controls.vi"("Control Label.Text Array"=w1154, "error in (no error)"=w1156, "VI ref"=w1157) -> ()  [unwired: 9 in]
          }
        }
      }
    }
  }
